vi "AutoBurn - BCU.vi"() -> ()   [LabVIEW 2018]
uses:
  <vilib>/Utility/config.llb/Read Key (String).vi
  <vilib>/Utility/config.llb/Write Key (String).vi
  <vilib>/Utility/file.llb/Read From Spreadsheet File (string).vi
  Settings/ControlCAN.dll
  <vilib>/Utility/config.llb/NI_LVConfig.lvlib
panel:
  out "?":bool
  in  "波特率 2":T1(ring)=enum."500Kbps"
  in  "错误输入（无错误）":errorcluster
  out "开始下载数据":u32
  out "开始下载数据":bool=TRUE
  out "耗时：":u32
  out "start":u32
  out "update flag":bool=TRUE
  in  "目标板类型":enum16{"BCU/主板", "BMU/从板"}(ring)
  out "Random":u32
  out "CRC16":u16 format="%x"
  out "进入烧录":bool
  out "boot模式应答计数":i32
  out "boot模式应答...成功":bool=TRUE
  out "总行数":i32
  in  "错误输入（无错误） 7":errorcluster caption="错误输入（无错误）"
  out "错误输出 18":errorcluster caption="错误输出"
  out "当前发送行":i32
  in  "错误输入（无错误） 6":errorcluster caption="错误输入（无错误）"
  out "错误输出 17":errorcluster caption="错误输出"
  in  "错误输入（无错误） 5":errorcluster caption="错误输入（无错误）"
  out "错误输出 16":errorcluster caption="错误输出"
  in  "错误输入（无错误） 4":errorcluster caption="错误输入（无错误）"
  out "错误输出 15":errorcluster caption="错误输出"
  in  "错误输入（无错误） 3":errorcluster caption="错误输入（无错误）"
  out "错误输出 14":errorcluster caption="错误输出"
  out "错误输出 13":errorcluster caption="错误输出"
  out "错误输出 12":errorcluster caption="错误输出"
  out "总电压":dbl
  out "Life":dbl
  out "返回类型":u32 format="%x"
  out "Info：":string
  in  "手动进入编程模式 2":bool
  out "T9":bool=TRUE
  out "T8":u8
  out "T7":bool=TRUE
  out "T6":bool=TRUE
  out "T5":bool=TRUE
  out "T4":bool=TRUE
  out "T3":bool=TRUE
  out "T2":bool=TRUE
  out "T1":bool=TRUE
  out "ID":u32 format="%x"
  out "错误输出 3":errorcluster caption="错误输出"
  in  "Monitor":bool
  out "校验":bool
  in  "请选择板号":u16(ring)=1 items=["BMU1"=1, "BMU2"=2, "BMU3"=3, "BMU4"=4, "BMU5"=5, "BMU6"=6, "BMU7"=7, "BMU8"=8, "BMU9"=9, "BMU10"=10, "BMU11"=11, "BMU12"=12, "BMU13"=13, "BMU14"=14, "BMU15"=15, "BMU16"=16, "BMU17"=17, "BMU18"=18, "BMU19"=19, "BMU20"=20]
  in  "手动进入编程模式":bool
  in  "板类型":enum16{"请选择板类型", "主板", "从板", "高压板"}(ring)=enum."主板"
  out "烧录结果":bool=TRUE
  out "擦除完成":bool
  out "进入烧录模式":bool
  out "MD5校验":bool
  out "进度":u8(slide) scale=0.0..100.0
  out "校验码实际值":string
  in  "校验码期望值":string
  in  "应用程序路径":path
  out "连接状态":bool=TRUE
  in  "类型":u32(ring)=4 items=["PCI5121"=1, "PCI9810"=2, "USBCAN1"=3, "USBCAN2"=4, "PCI9820"=5, "CAN232"=6, "PCI5110"=7, "CANLite(mini)"=8, "ISA9620"=9, "ISA5420"=10, "PC104CAN"=11, "CANET"=17, "DNP9810"=13, "USBCAN-E-U"=20, "USBCAN-2E-U"=21]
  in  "CAN路数":u32(ring) items=["0", "1"]
  in  "滤波方式":u8(ring) items=["Dual Filter", "Single Filter"]
  in  "工作方式":u8(ring) items=["Normal", "Listen Only"]
  in  "波特率":T1(ring)=enum."500Kbps"
  in  "设备索引":u32(ring) items=["0", "1", "2", "3", "4", "5", "6", "7", "8", "9", "10", "11", "12", "13", "14", "15", ""]
  in  "开始监控":bool
  out "CAN数据":bool
  out "Monitor_flag":bool
  out "PC端-协议类型 2":enum16{"TCP服务器Server", "TCP客户端Client"}(ring)
  out "通信端口:":u32
  out "CANET地址格式如：192.168.0.178":string
  out "发送数据长度":dbl
  out "发送的数据":i32[](array[numeric])
  in  "设备索引 4":u16(ring) items=["0", "1", "2", "3", "4", "5", "6", "7", "8", "9", "10", "11", "12", "13", "14", "15", ""]
  in  "CAN路数 4":u16(ring) items=["0", "1"]
  in  "设备类型 4":u16(ring)=4 items=["PCI5121"=1, "PCI9810"=2, "USBCAN1"=3, "USBCAN2"=4, "PCI9820"=5, "CAN232"=6, "PCI5110"=7, "CANLite(mini)"=8, "ISA9620"=9, "ISA5420"=10, "PC104CAN"=11, "CANETE"=12, "DNP9810"=13]
  out "Mode":bool
  in  "开始监控 2":bool
  out "大小":i32=426
  out "地址长度 2":u32=4
  out "数据长度 2":u32=64
  out "子字符串 2":string="9B2F9B349B399B3E9B439B499B4F9B559B5B9B619B679B6D9B739B799B7F7C7B"
  out "数据长度":u32=64
  out "地址长度":u32=4
  in  "设定":bool
  out "VCI_CAN_OBJ_T":T2 {"ID" format="%x"}
  out "子数组":string[](array[string])
  in  "从板号":dbl
  out "从板号2":dbl
  in  "读取":bool
  in  "停止 3":bool
  out "TEMP":bool
  out "CAN状态 2":bool
  out "VCI_CAN_OBJ_R":T2={"ID"=0, "TimeStamp"=0, "TimeFlag"=0, "SendType"=1, "RemoteFlag"=0, "ExternFlag"=0, "DataLen"=8, 0, 0, 0, 0, 0, 0, 0, 0, 0, 0, 0}
  in  "停止 2":bool
  out "接收":T2={"ID"=0, "TimeStamp"=61537964, "TimeFlag"=1, "SendType"=250, "RemoteFlag"=0, "ExternFlag"=0, "DataLen"=1, 255, 0, 0, 0, 0, 0, 0, 0, 0, 0, 124} {"ID" min=2 max=104373490 step=1 format="%x"; "TimeStamp" min=1962977793 max=3175728; "TimeFlag" min=1 max=0; "SendType" max=131 step=11; "RemoteFlag" min=52 max=6 step=1; "ExternFlag" max=0; "DataLen" min=1 max=170; "?" min=117 max=48 step=117; "?" min=48 max=0; "?" max=0; "?" min=2 max=0; "?" max=150 step=11; "?" min=52 max=6 step=1; "?" max=0; "?" min=1 max=170; "?" min=120 max=175; "?" max=12; "?" max=0}
  out "收到请求":bool=TRUE
  out "分配":bool
  out "设置中？ 2":bool
  in  "Boar_Type":bool
  out "temp1":bool
  out "设置中？":bool
  in  "总步骤":dbl=21.0
  in  "失败重测次数":dbl=3.0
  out "一键测试":bool
  out "测试结果":bool
  in  "行号":dbl=21.0
  in  "工作方式 2":u8(ring) items=["Normal", "Listen Only"]
  in  "设备类型 2":u16(ring)=4 items=["PCI5121"=1, "PCI9810"=2, "USBCAN1"=3, "USBCAN2"=4, "PCI9820"=5, "CAN232"=6, "PCI5110"=7, "CANLite(mini)"=8, "ISA9620"=9, "ISA5420"=10, "PC104CAN"=11, "CANETE"=12, "DNP9810"=13]
  in  "停止":bool
  out "CAN状态":bool=TRUE
  in  "监控":bool
  # "当前BMU信息"
  # "BootLoader_V1.0.0"
  # "注意：升级完成后系统需要重新上电才能正常运行！"
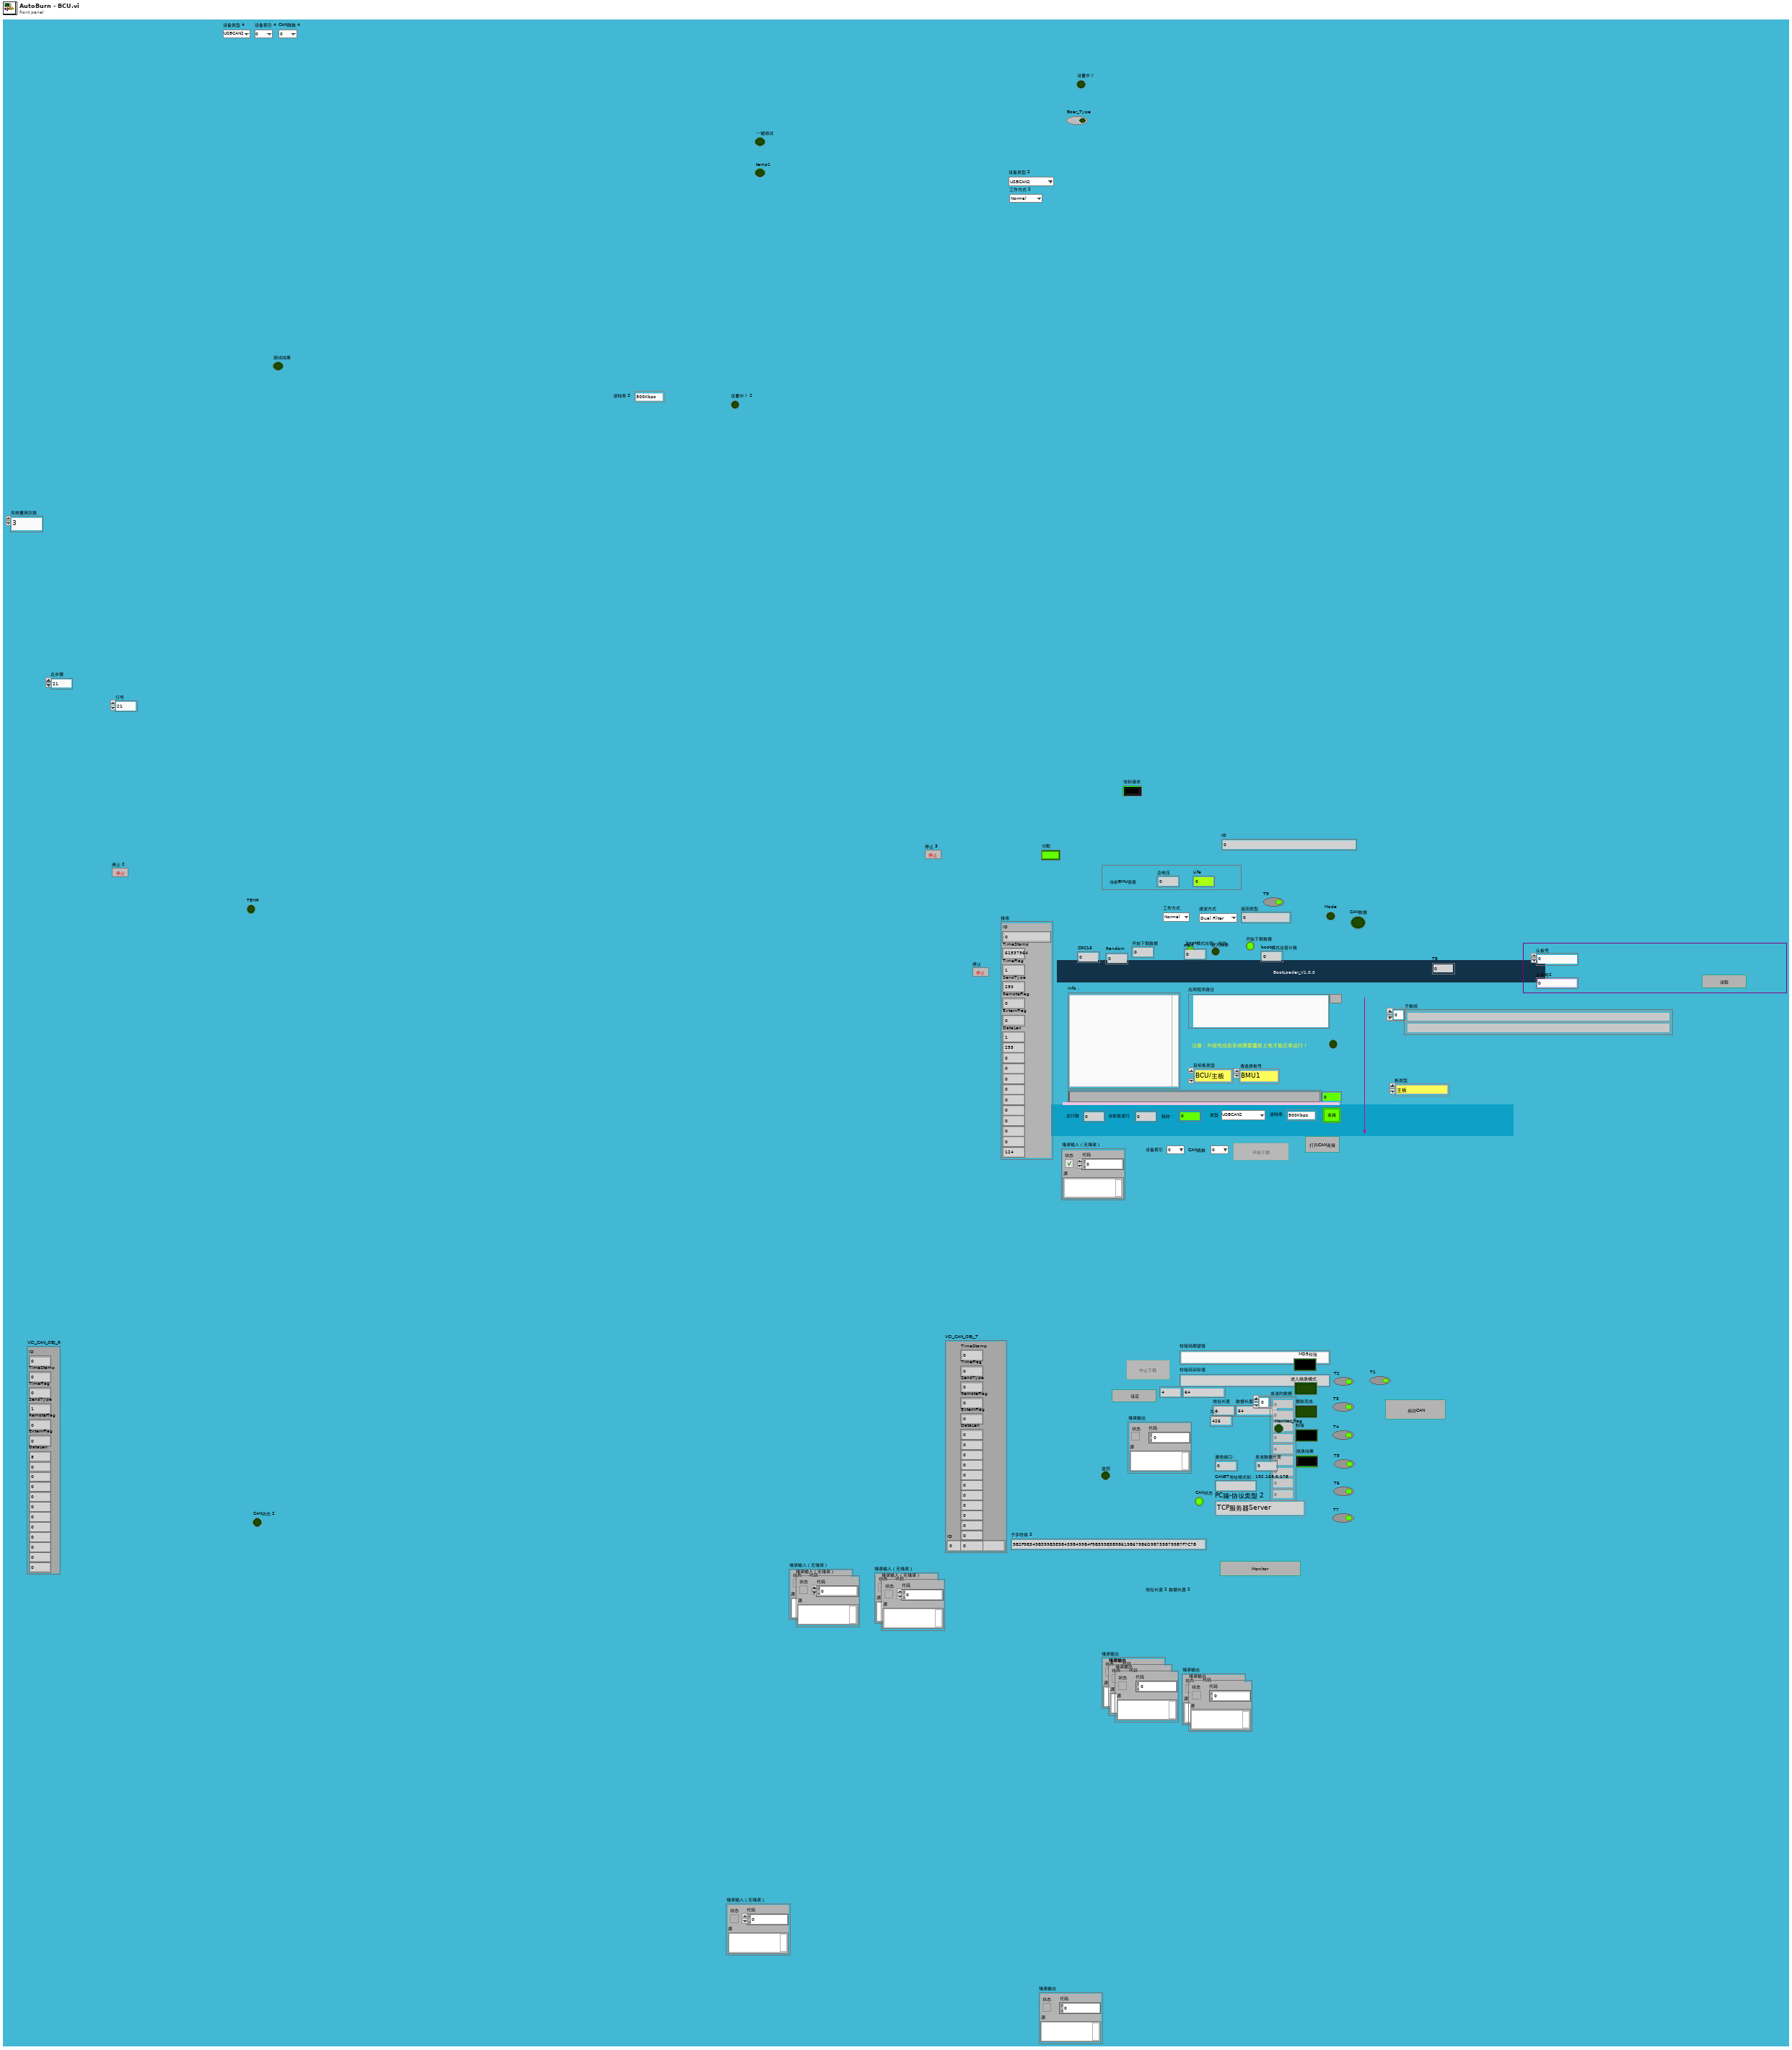
[diagram p1: front panel]
types:
  T1 = enum16{"5Kbps", "10Kbps", "20Kbps", "40Kbps", "50Kbps", "80Kbps", "100Kbps", "125Kbps", "200Kbps", "250Kbps", "400Kbps", "500Kbps", "666Kbps", "800Kbps", "1000Kbps"}
  T2 = cluster{"ID":u32, "TimeStamp":u32, "TimeFlag":u8, "SendType":u8, "RemoteFlag":u8, "ExternFlag":u8, "DataLen":u8, u8, u8, u8, u8, u8, u8, u8, u8, u8, u8, u8}
  T3 = enum8{"Enabled", "Disabled", "Disabled and Grayed Out"}
  T4 = typedef "NI_LVConfig.lvlib/Config Data RefNum.ctl" = refnum<k1>
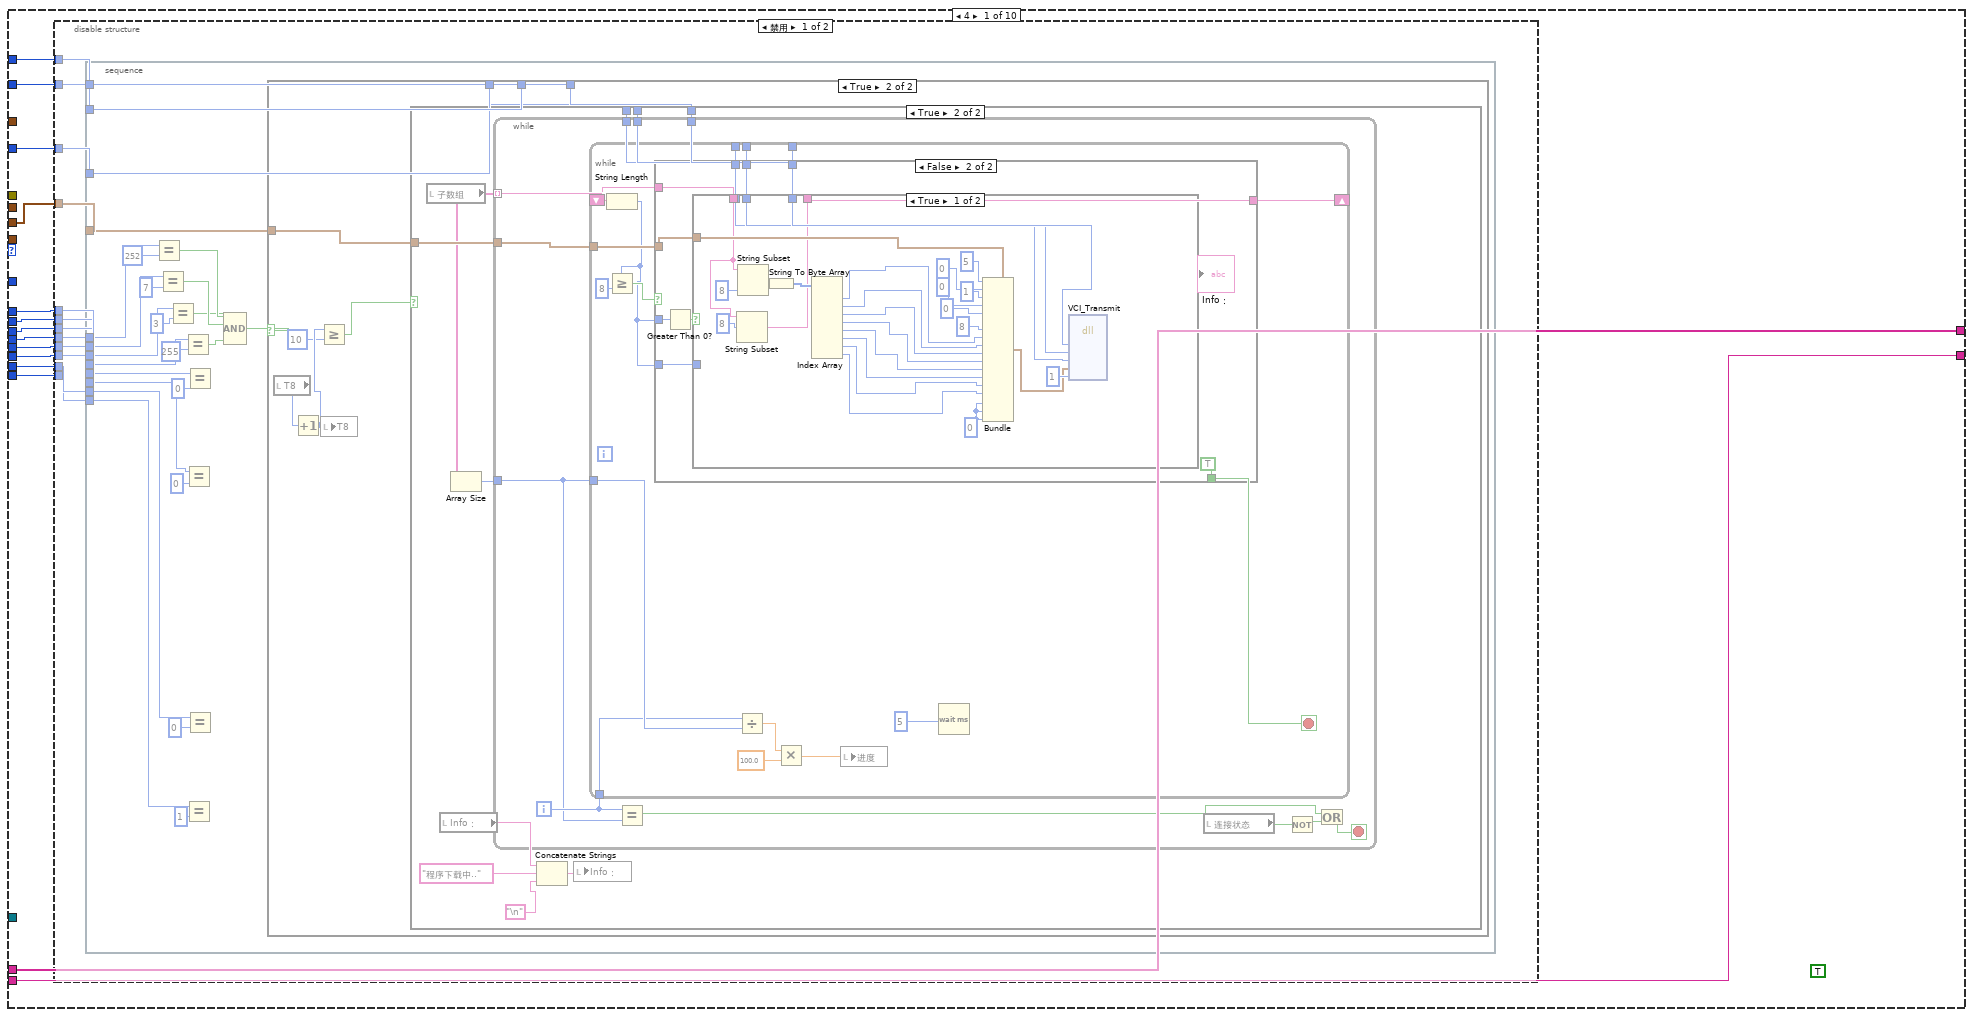
[diagram p3: hidden frame]
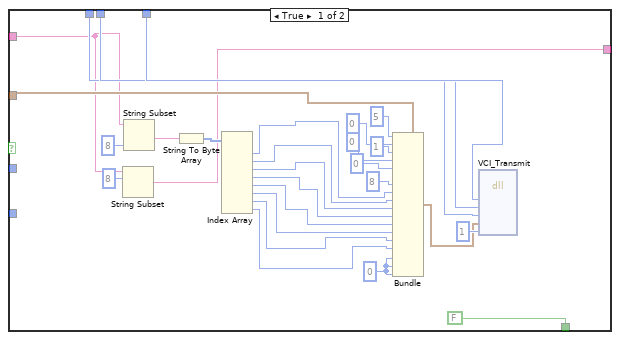
[diagram p6: hidden frame]
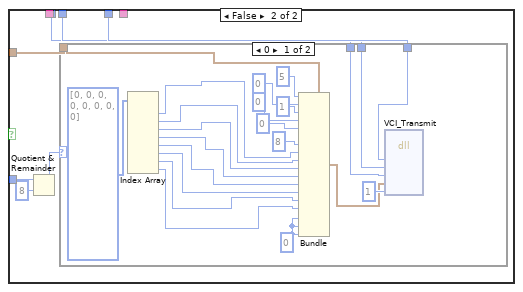
[diagram p7: hidden frame]
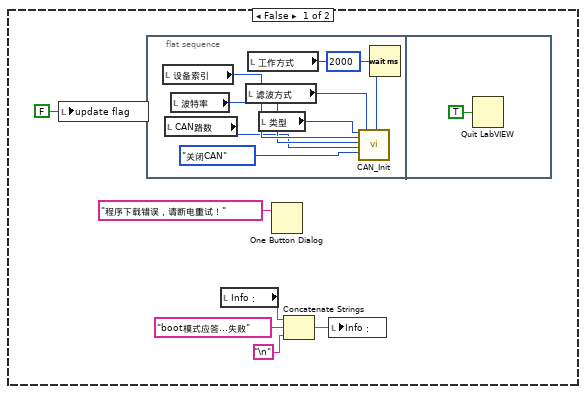
[diagram p10: hidden frame]
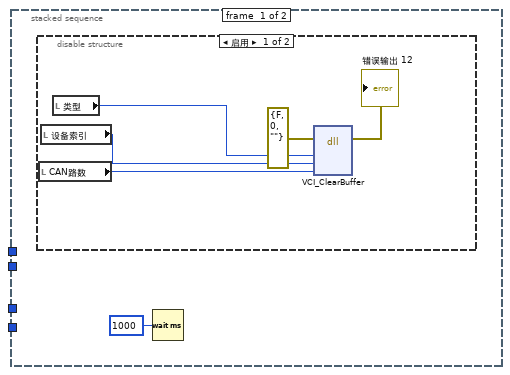
[diagram p11: hidden frame]
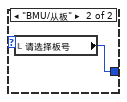
[diagram p13: hidden frame]
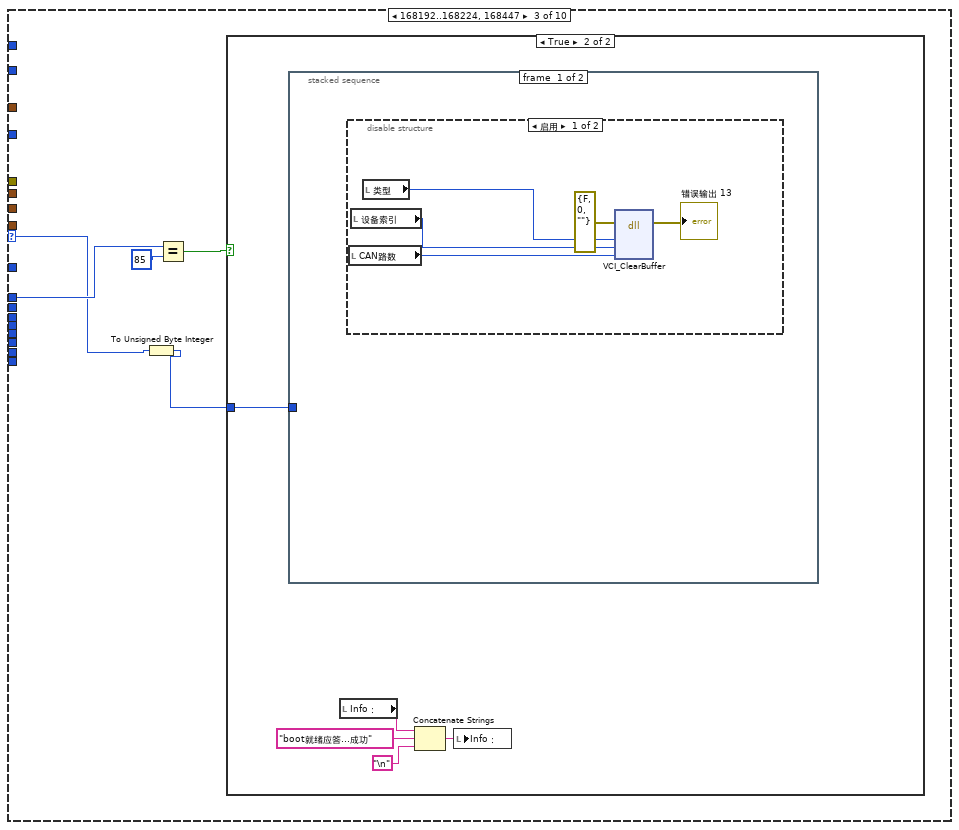
[diagram p14: hidden frame]
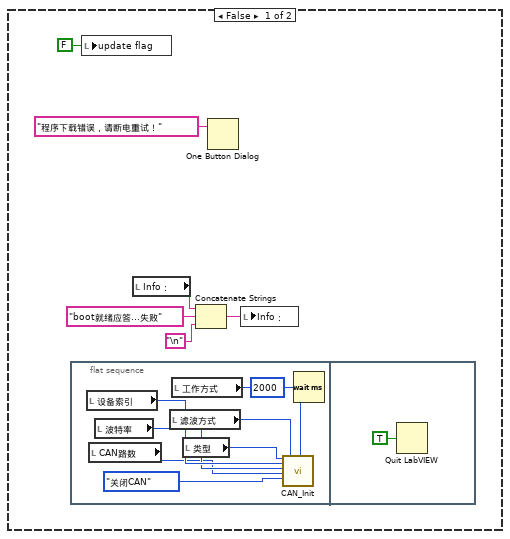
[diagram p15: hidden frame]
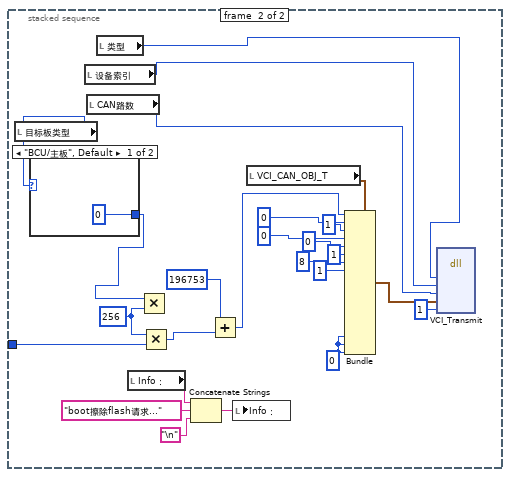
[diagram p17: hidden frame]
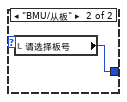
[diagram p18: hidden frame]
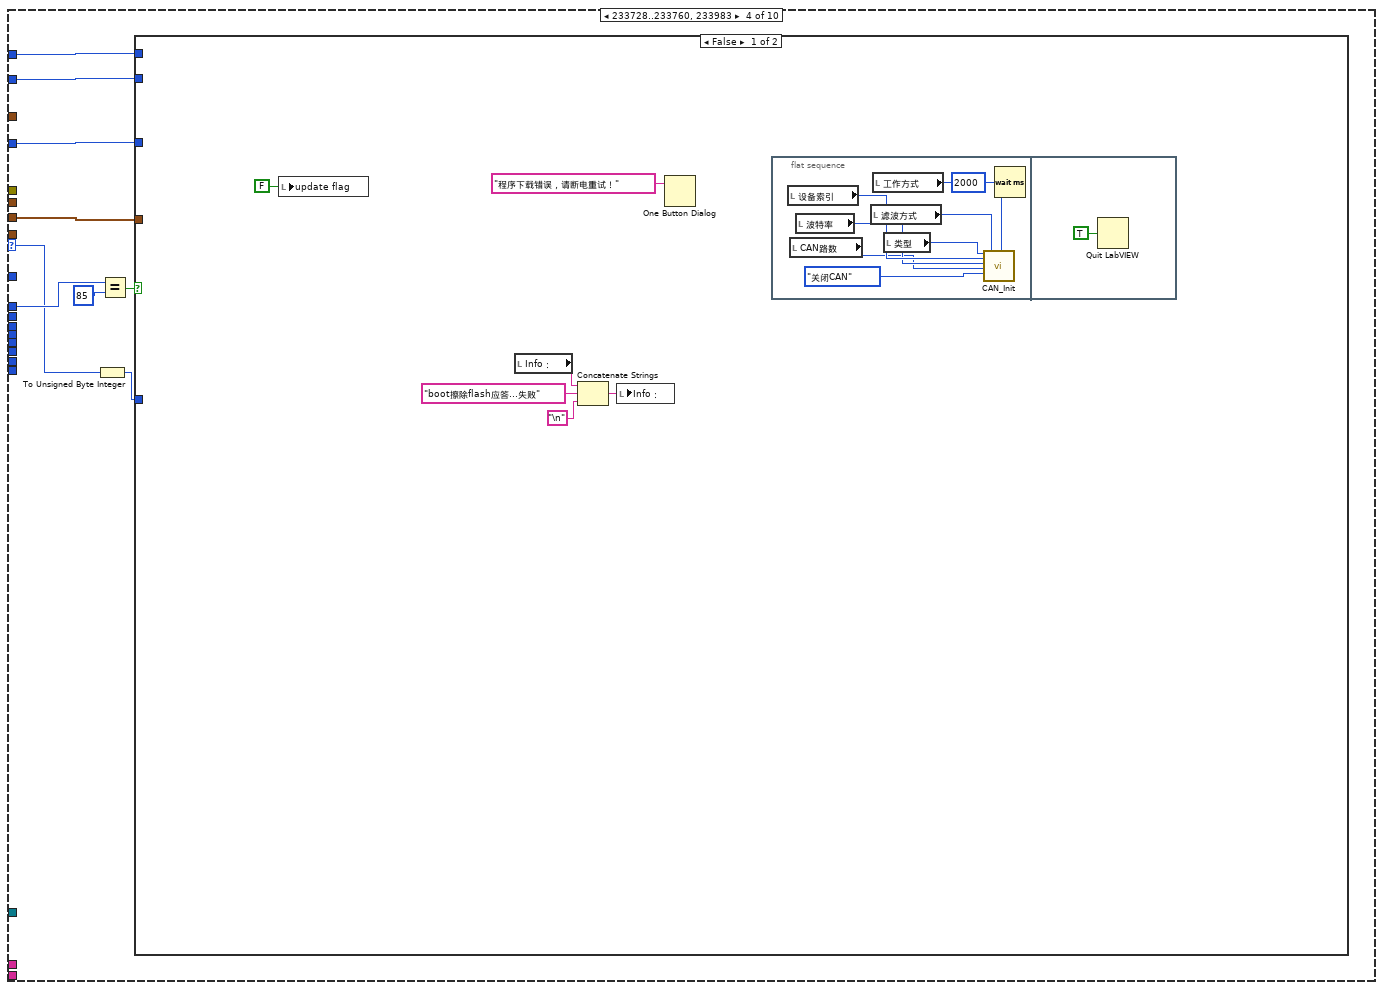
[diagram p19: hidden frame]
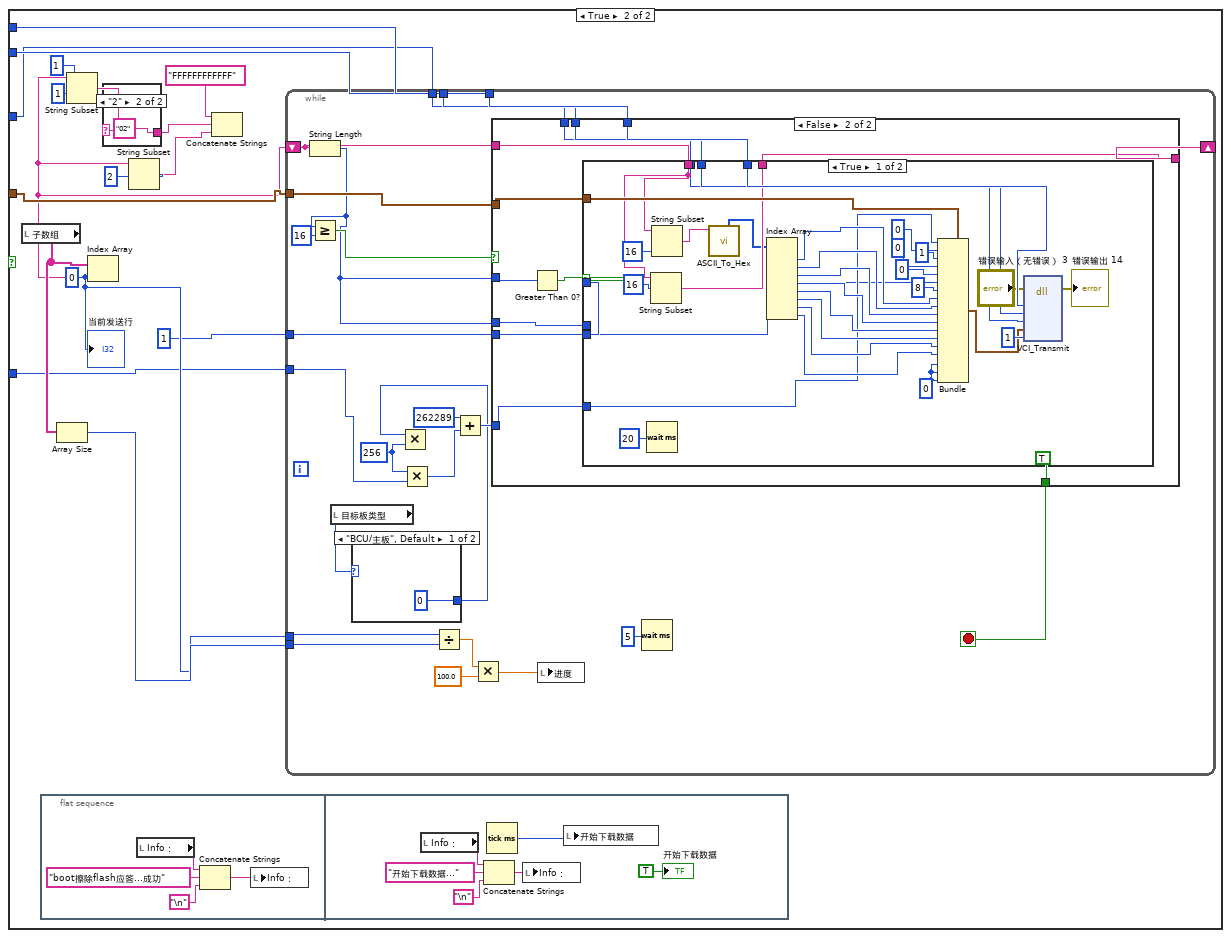
[diagram p20: hidden frame]
diagram:
  (unwired) u32 0
  (unwired) u32 255
  w21 = "" ("布尔文本.文本")
  w22 = cluster{u32, u32}[] [{0, 0}] ("颜色[4]")
  w29 = "" ("校验码期望值")
  w37 = FALSE ("进入烧录模式")
  n1 = local write "TEMP"(FALSE ("TEMP")) -> ()
  n2 = local read "VCI_CAN_OBJ_R"() -> (w19:T2)
  n3 = local write "校验码期望值"(w29) -> ()
  n4 = local write "校验码实际值"(w29) -> ()
  n5 = property on="校验" class="Bool (strict)"("Colors [4]"=w22, "BoolText.Text"=w21) -> ()  [unwired: 2 in, 2 out]
  n6 = Obtain Queue(name (unnamed)="CAN1" ("名称（未命名）"), element data type=w19, error in (no error)="错误输入（无错误）") -> (queue out=w20:refnum<queue>, error out=w7:errorcluster)  [unwired: 2 in, 1 out]
  n7 = property on="烧录结果" class="Bool (strict)"("Colors [4]"=w22, "BoolText.Text"=w21) -> ()  [unwired: 2 in, 2 out]
  n8 = Initialize Array("", 1 ("维数大小")) -> (w33:string[])
  n9 = local write "连接状态"(FALSE ("连接状态")) -> ()
  n10 = local write "boot模式应答...成功"(FALSE ("boot模式应答...成功")) -> ()
  n11 = local write "开始下载数据"(u32 0 ("开始下载数据")) -> ()
  n12 = local write "耗时："(u32 0 ("耗时：")) -> ()
  n13 = property on="请选择板号" class="Ring (strict)"("Visible"=TRUE ("可见")) -> ()  [unwired: 2 in, 2 out]
  n14 = local write "耗时："(u32 0 ("耗时：")) -> ()
  n15 = while {
    tunnel: w20 -> [w44]
    shift-right: [w47] -> _
    shift-left: w33 -> [w48]
    shift-right: [w45] -> _
    shift-left: "" -> [w46]
    tunnel: w7 -> [w43]
    stop <- "停止 3" stop-if-true
    n16 = local read "update flag"() -> (w40:bool)
    n17 = Dequeue Element(queue=w44, error in (no error)=w43) -> (element=w41:T2, error out=w42:errorcluster)  [unwired: 1 in, 2 out]
    n18 = case shown="True" w40 {
      tunnel: w48 -> [_ w67]
      tunnel: [_ w66] -> w47
      tunnel: w46 -> [_ w65]
      tunnel: [_ w64] -> w45
      tunnel: w44 -> [_ w62]
      tunnel: w42 -> [_ w61]
      tunnel: w41 -> [_ w60]
      frame False {
      }
      frame True {
        n19 = local read "VCI_CAN_OBJ_T"() -> (w70:T2)
        n20 = local read "CAN路数"() -> (w68:u32)
        n21 = Unbundle(w60) -> ("ID"=w59:u32, w58:u8, w57:u8, w56:u8, w55:u8, w54:u8, w53:u8, w52:u8, w51:u8)  [unwired: 9 out]
        n22 = local read "类型"() -> (w69:u32)
        n23 = local read "设备索引"() -> (w50:u32)
        n24 = case shown="19100..19120, 191FF" w59 {
          selector: w59 -> [_ w266 w348 w404 w592 _ _ _ _ w1335]
          tunnel: w60 -> [_ _ _ _ _ _ _ _ _ _]
          tunnel: w70 -> [w84 _ _ w408 w596 w814 w879 _ w1115 _]
          tunnel: w69 -> [w83 _ _ w407 w595 w813 w881 w1009 w1123 _]
          tunnel: w50 -> [w82 _ _ w406 w594 w812 w880 w1008 w1122 _]
          tunnel: w68 -> [w81 _ _ w405 w593 w811 w878 w1007 w1121 _]
          tunnel: w67 -> [w80 _ _ _ _ w810 w883 w1006 w1117 w1337]
          tunnel: [w80 _ _ _ _ w810 w882 w1006 w1118 w1337] -> w66
          tunnel: w65 -> [w79 _ _ _ _ w809 w877 w1011 w1119 w1336]
          tunnel: [w79 _ _ _ _ w809 w876 w1010 w1120 w1336] -> w64
          tunnel: "板类型" -> [_ _ _ _ _ _ w875 w1005 w1116 _]
          tunnel: w62 -> [_ _ _ _ _ w808 w874 w1004 w1114 _]
          tunnel: w61 -> [_ _ _ _ _ _ _ _ _ _]
          tunnel: w60 -> [_ _ _ _ _ _ _ w995 _ _]
          tunnel: w60 -> [_ _ _ _ _ _ _ _ w1113 _]
          tunnel: w58 -> [w78 w269 w350 w411 _ _ _ _ _ _]
          tunnel: w57 -> [w77 w264 _ _ _ _ _ _ _ _]
          tunnel: w56 -> [w76 w263 _ _ w590 _ _ _ _ _]
          tunnel: w55 -> [w75 w262 _ _ _ _ _ _ _ _]
          tunnel: w54 -> [w74 w261 _ _ _ _ _ _ _ _]
          tunnel: w53 -> [w73 _ _ _ _ _ _ _ _ _]
          tunnel: w52 -> [w72 _ _ _ _ _ _ _ _ w1331]
          tunnel: w51 -> [w71 _ _ _ _ _ _ _ _ w1330]
          frame 4 {
            (unwired) TRUE
            n25 = disable-structure shown="禁用" {
              disable-tunnel: w84 -> [w96 _]
              disable-tunnel: w83 -> [w95 _]
              disable-tunnel: w82 -> [w94 _]
              disable-tunnel: w81 -> [w93 _]
              disable-tunnel: w78 -> [w92 _]
              disable-tunnel: w77 -> [w91 _]
              disable-tunnel: w76 -> [w90 _]
              disable-tunnel: w75 -> [w89 _]
              disable-tunnel: w74 -> [w88 _]
              disable-tunnel: w73 -> [w87 _]
              disable-tunnel: w72 -> [w86 _]
              disable-tunnel: w71 -> [w85 _]
              frame Disabled {
                n26 = stacked-sequence {
                  tunnel: w96 -> [w121]
                  tunnel: w95 -> [w120]
                  tunnel: w94 -> [w119]
                  tunnel: w93 -> [w118]
                  tunnel: w92 -> [w117]
                  tunnel: w91 -> [w116]
                  tunnel: w90 -> [w115]
                  tunnel: w89 -> [w114]
                  tunnel: w88 -> [w113]
                  tunnel: w87 -> [w112]
                  tunnel: w86 -> [w111]
                  tunnel: w85 -> [w110]
                  frame #0 {
                    n27 = Equal?(x=w117, y=u8 252) -> (x = y?=w101:bool)
                    n28 = Equal?(x=w116, y=u8 7) -> (x = y?=w100:bool)
                    n29 = Equal?(x=w115, y=u8 3) -> (x = y?=w99:bool)
                    n30 = Equal?(x=w114, y=u8 255) -> (x = y?=w98:bool)
                    n31 = Equal?(x=w112, y=u8 0) -> ()  [unwired: 1 out]
                    n32 = Equal?(x=w110, y=u8 1) -> ()  [unwired: 1 out]
                    n33 = Equal?(x=w113, y=u8 0) -> ()  [unwired: 1 out]
                    n34 = Equal?(x=w111, y=u8 0) -> ()  [unwired: 1 out]
                    n35 = Compound Arithmetic op=AND(w101, w100, w99, w98) -> (w97:bool)
                    n36 = case shown="True" w97 {
                      tunnel: w121 -> [_ w129]
                      tunnel: w120 -> [_ w128]
                      tunnel: w119 -> [_ w127]
                      tunnel: w118 -> [_ w126]
                      frame False {
                      }
                      frame True {
                        n37 = local read "T8"() -> (w125:u8)
                        n38 = Increment(x=w125) -> (x+1=w124:u8)
                        n39 = Greater Or Equal?(x=w124, y=u8 10) -> (x >= y?=w122:bool)
                        n40 = local write "T8"(w124) -> ()
                        n41 = case shown="True" w122 {
                          tunnel: w129 -> [_ w139]
                          tunnel: w128 -> [_ w138]
                          tunnel: w127 -> [_ w137]
                          tunnel: w126 -> [_ w136]
                          frame False {
                          }
                          frame True {
                            n42 = local read "子数组"() -> (w135:string[])
                            n43 = local read "Info："() -> (w131:string)
                            n44 = Array Size(array=w135) -> (size(s)=w134:i32)
                            n45 = while {
                              tunnel: w139 -> [w150]
                              tunnel: w138 -> [w149]
                              tunnel: w137 -> [w148]
                              tunnel: w136 -> [w147]
                              tunnel: w135 -> [w146] mode=indexing
                              tunnel: w134 -> [w143]
                              i -> [w144]
                              stop <- w142 stop-if-true
                              n46 = while {
                                tunnel: w150 -> [w166]
                                tunnel: w149 -> [w165]
                                tunnel: w148 -> [w164]
                                tunnel: w147 -> [w163]
                                shift-right: [w158] -> _
                                shift-left: w146 -> [w159]
                                tunnel: w143 -> [w156]
                                tunnel: w144 -> [w152]
                                stop <- w151 stop-if-true
                                n47 = String Length(string=w159) -> (length=w157:i32)
                                n48 = Greater Or Equal?(x=w157, y=8) -> (x >= y?=w160:bool)
                                n49 = case shown="False" w160 {
                                tunnel: w166 -> [w194 w204]
                                tunnel: w165 -> [w193 w203]
                                tunnel: w164 -> [w192 w202]
                                tunnel: w163 -> [w191 w201]
                                tunnel: w159 -> [w180 w200]
                                tunnel: [w168 w199] -> w158
                                tunnel: [FALSE TRUE] -> w151
                                tunnel: w157 -> [_ w197]
                                tunnel: w157 -> [_ w195]
                                frame True {
                                w187 = u8 0 ("元素")
                                n50 = String Subset(string=w180, offset (0)=8 ("偏移量(0)")) -> (substring=w168:string)  [unwired: 1 in]
                                n51 = String Subset(string=w180, length (rest)=8 ("长度（剩余）")) -> (substring=w178:string)  [unwired: 1 in]
                                n52 = String To Byte Array(string=w178) -> (unsigned byte array=w177:u8[])
                                n53 = Index Array(array=w177) -> (element #1=w176:u8, element #2=w175:u8, element #3=w174:u8, element #4=w173:u8, element #5=w172:u8, element #6=w171:u8, element #7=w170:u8, element #8=w169:u8)  [unwired: 8 in]
                                n54 = Bundle(cluster=w194, "ID"=u32 5, "TimeStamp"=u8 0 ("RemoteFlag"), "TimeFlag"=u8 1, "SendType"=u8 0 ("DataLen"), "RemoteFlag"=u8 0, "DataLen"=u8 8, w176, w175, w174, w173, w172, w171, w170, w169, w187, w187, w187) -> (w182:T2)  [unwired: 1 in]
                                n55 = dll-call lib="PTH2{abs DPCTools2.sourceSNV-AutoTestV1.0.0ASettingsSEQEditDriver平台BCUAutoBurnSettingsControlCAN.dll" fn="VCI_Transmit"("DeviceType"=w193, "DeviceInd"=w192, "CANInd"=w191, "pSend"=w182, "Len"=u32 1) -> ()  [unwired: 5 in, 6 out]
                                }
                                frame False {
                                n56 = Greater Than 0?(x=w197) -> (x > 0?=w196:bool)
                                n57 = case shown="True" w196 {
                                tunnel: w204 -> [w231 w238]
                                tunnel: w203 -> [w230 w237]
                                tunnel: w202 -> [w229 w236]
                                tunnel: w201 -> [w228 w235]
                                tunnel: w200 -> [w217 _]
                                tunnel: [w206 _] -> w199
                                tunnel: w195 -> [_ w233]
                                frame True {
                                w224 = u8 0 ("元素")
                                n58 = String Subset(string=w217, offset (0)=8 ("偏移量(0)")) -> (substring=w206:string)  [unwired: 1 in]
                                n59 = String Subset(string=w217, length (rest)=8 ("长度（剩余）")) -> (substring=w216:string)  [unwired: 1 in]
                                n60 = String To Byte Array(string=w216) -> (unsigned byte array=w215:u8[])
                                n61 = Index Array(array=w215) -> (element #1=w214:u8, element #2=w213:u8, element #3=w212:u8, element #4=w211:u8, element #5=w210:u8, element #6=w209:u8, element #7=w208:u8, element #8=w207:u8)  [unwired: 8 in]
                                n62 = Bundle(cluster=w231, "ID"=u32 5, "TimeStamp"=u8 0 ("RemoteFlag"), "TimeFlag"=u8 1, "SendType"=u8 0 ("DataLen"), "RemoteFlag"=u8 0, "DataLen"=u8 8, w214, w213, w212, w211, w210, w209, w208, w207, w224, w224, w224) -> (w219:T2)  [unwired: 1 in]
                                n63 = dll-call lib="PTH2{abs DPCTools2.sourceSNV-AutoTestV1.0.0ASettingsSEQEditDriver平台BCUAutoBurnSettingsControlCAN.dll" fn="VCI_Transmit"("DeviceType"=w230, "DeviceInd"=w229, "CANInd"=w228, "pSend"=w219, "Len"=u32 1) -> ()  [unwired: 5 in, 6 out]
                                }
                                frame False {
                                n64 = Quotient & Remainder(x=w233, y=8) -> (x-y*floor(x/y)=w232:i32)  [unwired: 1 out]
                                n65 = case shown="0" w232 {
                                tunnel: w238 -> [w260 _]
                                tunnel: w237 -> [w259 _]
                                tunnel: w236 -> [w258 _]
                                tunnel: w235 -> [w257 _]
                                frame 0 {
                                w253 = u8 0 ("元素")
                                n66 = Index Array(array=u8[] [0, 0, 0, 0, 0, 0, 0, 0] ("数组")) -> (element #1=w247:u8, element #2=w246:u8, element #3=w245:u8, element #4=w244:u8, element #5=w243:u8, element #6=w242:u8, element #7=w241:u8, element #8=w240:u8)  [unwired: 8 in]
                                n67 = Bundle(cluster=w260, "ID"=u32 5, "TimeStamp"=u8 0 ("RemoteFlag"), "TimeFlag"=u8 1, "SendType"=u8 0 ("DataLen"), "RemoteFlag"=u8 0, "DataLen"=u8 8, w247, w246, w245, w244, w243, w242, w241, w240, w253, w253, w253) -> (w248:T2)  [unwired: 1 in]
                                n68 = dll-call lib="PTH2{abs DPCTools2.sourceSNV-AutoTestV1.0.0ASettingsSEQEditDriver平台BCUAutoBurnSettingsControlCAN.dll" fn="VCI_Transmit"("DeviceType"=w259, "DeviceInd"=w258, "CANInd"=w257, "pSend"=w248, "Len"=u32 1) -> ()  [unwired: 5 in, 6 out]
                                }
                                frame 1, Default {
                                }
                                }
                                }
                                }
                                }
                                }
                                n69 = Divide(x=w152, y=w156) -> (x/y=w155:dbl)
                                n70 = Multiply(x=w155, y=100.0) -> (x*y=w153:dbl)
                                n71 = local write "进度"(w153) -> ()
                                n72 = Wait (ms)(milliseconds to wait=u32 5 ("等待时间（毫秒）")) -> ()  [unwired: 1 out]
                              }
                              n73 = Equal?(x=w144, y=w143) -> (x = y?=w140:bool)
                              n74 = local read "连接状态"() -> (w145:bool)
                              n75 = Not(x=w145) -> (.not. x?=w141:bool)
                              n76 = Or(x=w140, y=w141) -> (x .or. y?=w142:bool)
                            }
                            n77 = Concatenate Strings(w131, "程序下载中.." ("字符串"), "\n") -> (w130:string)
                            n78 = local write "Info："(w130) -> ()
                          }
                        }
                      }
                    }
                  }
                }
              }
              frame Enabled {
              }
            }
          }
          frame 102656..102688, 102911 {
            n79 = To Unsigned Byte Integer(number=w266) -> (unsigned 8bit integer=w265:u8)
            n80 = Equal?(x=w269, y=u8 85) -> (x = y?=w268:bool)
            n81 = case shown="True" w268 {
              tunnel: w265 -> [_ w301]
              tunnel: w264 -> [_ w298]
              tunnel: w263 -> [_ w296]
              tunnel: w262 -> [_ w297]
              tunnel: w261 -> [_ w295]
              frame False {
                n82 = local write "update flag"(FALSE ("update flag")) -> ()
                n83 = flat-sequence {
                  frame #0 {
                    n84 = local read "设备索引"() -> (w282:u32)
                    n85 = local read "CAN路数"() -> (w280:u32)
                    n86 = local read "波特率"() -> (w281:T1)
                    n87 = local read "滤波方式"() -> (w279:u8)
                    n88 = local read "工作方式"() -> (w278:u8)
                    n89 = local read "类型"() -> (w283:u32)
                    n90 = call "CAN_Init.vi"("设备类型"=w283, "设备索引"=w282, "波特率"=w281, "CAN路数"=w280, "操作类型"=enum16{"初始化CAN", "关闭CAN"}."关闭CAN", "滤波方式"=w279, "工作方式"=w278) -> ()  [unwired: 11 in, 2 out]
                    n91 = Wait (ms)(milliseconds to wait=u32 2000 ("等待时间（毫秒）")) -> ()  [unwired: 1 out]
                  }
                  frame #1 {
                    n92 = Quit LabVIEW(quit? (T)=TRUE ("退出？(T)")) -> ()
                  }
                }
                n93 = local read "Info："() -> (w272:string)
                n94 = One Button Dialog(message="程序下载错误，请断电重试！" ("消息")) -> ()  [unwired: 1 in, 1 out]
                n95 = Concatenate Strings(w272, "boot模式应答...失败" ("字符串"), "\n") -> (w275:string)
                n96 = local write "Info："(w275) -> ()
              }
              frame True {
                n97 = Join Numbers(hi=w298, lo=w297) -> ((hi.lo)=w294:u16)
                n98 = Join Numbers(hi=w295, lo=w296) -> ((hi.lo)=w293:u16)
                n99 = Join Numbers(hi=w294, lo=w293) -> ((hi.lo)=w292:u32)
                n100 = Not(x=w292) -> (.not. x?=w291:u32)
                "Random" <- w291
                n101 = Split Number(x=w291) -> (hi(x)=w290:u16, lo(x)=w289:u16)
                n102 = Split Number(x=w290) -> (hi(x)=w288:u8, lo(x)=w287:u8)
                n103 = Split Number(x=w289) -> (hi(x)=w286:u8, lo(x)=w285:u8)
                n104 = stacked-sequence {
                  tunnel: w301 -> [_ w322]
                  tunnel: w288 -> [_ w317]
                  tunnel: w287 -> [_ w316]
                  tunnel: w286 -> [_ w315]
                  tunnel: w285 -> [_ w314]
                  frame #0 {
                    n105 = disable-structure shown="启用" {
                      frame Enabled {
                        n106 = local read "CAN路数"() -> (w309:u32)
                        n107 = local read "设备索引"() -> (w310:u32)
                        n108 = local read "类型"() -> (w311:u32)
                        n109 = dll-call lib="PTH2{abs DPCTools2.sourceSNV-AutoTestV1.0.0ASettingsSEQEditDriver平台BCUAutoBurnSettingsControlCAN.dll" fn="VCI_ClearBuffer" label="VCI_Clearbuffer"(error in=errorcluster {"status"=FALSE, "code"=0, "source"=""} ("错误输入（无错误）"), "DeviceType"=w311, "DeviceInd"=w310, "CANInd"=w309) -> (error out=→"错误输出 12":errorcluster)  [unwired: 3 in, 4 out]
                      }
                      frame Disabled {
                      }
                    }
                    n110 = Wait (ms)(milliseconds to wait=u32 1000 ("等待时间（毫秒）")) -> ()  [unwired: 1 out]
                  }
                  frame #1 {
                    w323 = u16 256 ("y")
                    w338 = u8 0 ("元素")
                    n111 = local read "目标板类型"() -> (w313:enum16{"BCU/主板", "BMU/从板"})
                    n112 = case shown="\"BCU/主板\", Default" w313 {
                      tunnel: [u16 0 ("请选择板号") w345] -> w312
                      frame "BCU/主板", Default {
                      }
                      frame "BMU/从板" {
                        n113 = local read "请选择板号"() -> (w345:u16)
                      }
                    }
                    n114 = local read "设备索引"() -> (w333:u32)
                    n115 = local read "CAN路数"() -> (w332:u32)
                    n116 = local read "类型"() -> (w334:u32)
                    n117 = Multiply(x=w312, y=w323) -> ()  [unwired: 1 out]
                    n118 = Multiply(x=w323, y=w322) -> (x*y=w321:u16)
                    n119 = local read "Info："() -> (w327:string)
                    n120 = Add(x=u32 131217 ("ID"), y=w321) -> (x+y=w328:u32)
                    n121 = local read "VCI_CAN_OBJ_T"() -> (w331:T2)
                    n122 = local read "CRC16"() -> (w320:u16)
                    n123 = Concatenate Strings(w327, "boot就绪查询..." ("字符串"), "\n") -> (w324:string)
                    n124 = Split Number(x=w320) -> (hi(x)=w318:u8, lo(x)=w319:u8)
                    n125 = local write "Info："(w324) -> ()
                    n126 = Bundle(cluster=w331, "ID"=w328, "TimeStamp"=u8 0 ("RemoteFlag"), "TimeFlag"=u8 1, "SendType"=u8 0 ("DataLen"), "RemoteFlag"=u8 0, "ExternFlag"=u8 1, "DataLen"=u8 8, u8 1 ("元素"), w317, w316, w315, w314, w318, w319, w338, w338, w338) -> (w335:T2)  [unwired: 1 in]
                    n127 = dll-call lib="PTH2{abs DPCTools2.sourceSNV-AutoTestV1.0.0ASettingsSEQEditDriver平台BCUAutoBurnSettingsControlCAN.dll" fn="VCI_Transmit"("DeviceType"=w334, "DeviceInd"=w333, "CANInd"=w332, "pSend"=w335, "Len"=u32 1) -> ()  [unwired: 5 in, 6 out]
                  }
                }
                n128 = local read "Info："() -> (w302:string)
                n129 = local write "进入烧录"(FALSE ("进入烧录")) -> ()
                n130 = Concatenate Strings(w302, "boot模式应答...成功" ("字符串"), "\n") -> (w305:string)
                n131 = local write "Info："(w305) -> ()
                "boot模式应答...成功" <- TRUE
              }
            }
          }
          frame 168192..168224, 168447 {
            n132 = To Unsigned Byte Integer(number=w348) -> (unsigned 8bit integer=w347:u8)
            n133 = Equal?(x=w350, y=u8 85) -> (x = y?=w346:bool)
            n134 = case shown="True" w346 {
              tunnel: w347 -> [_ w370]
              frame False {
                n135 = flat-sequence {
                  frame #0 {
                    n136 = local read "设备索引"() -> (w363:u32)
                    n137 = local read "CAN路数"() -> (w361:u32)
                    n138 = local read "波特率"() -> (w362:T1)
                    n139 = local read "滤波方式"() -> (w360:u8)
                    n140 = local read "工作方式"() -> (w359:u8)
                    n141 = local read "类型"() -> (w364:u32)
                    n142 = call "CAN_Init.vi"("设备类型"=w364, "设备索引"=w363, "波特率"=w362, "CAN路数"=w361, "操作类型"=enum16{"初始化CAN", "关闭CAN"}."关闭CAN", "滤波方式"=w360, "工作方式"=w359) -> ()  [unwired: 11 in, 2 out]
                    n143 = Wait (ms)(milliseconds to wait=u32 2000 ("等待时间（毫秒）")) -> ()  [unwired: 1 out]
                  }
                  frame #1 {
                    n144 = Quit LabVIEW(quit? (T)=TRUE ("退出？(T)")) -> ()
                  }
                }
                n145 = local write "update flag"(FALSE ("update flag")) -> ()
                n146 = local read "Info："() -> (w353:string)
                n147 = Concatenate Strings(w353, "boot就绪应答...失败" ("字符串"), "\n") -> (w356:string)
                n148 = One Button Dialog(message="程序下载错误，请断电重试！" ("消息")) -> ()  [unwired: 1 in, 1 out]
                n149 = local write "Info："(w356) -> ()
              }
              frame True {
                n150 = stacked-sequence {
                  tunnel: w370 -> [_ w379]
                  frame #0 {
                    n151 = disable-structure shown="启用" {
                      frame Enabled {
                        n152 = local read "CAN路数"() -> (w373:u32)
                        n153 = local read "设备索引"() -> (w374:u32)
                        n154 = local read "类型"() -> (w375:u32)
                        n155 = dll-call lib="PTH2{abs DPCTools2.sourceSNV-AutoTestV1.0.0ASettingsSEQEditDriver平台BCUAutoBurnSettingsControlCAN.dll" fn="VCI_ClearBuffer" label="VCI_Clearbuffer"(error in=errorcluster {"status"=FALSE, "code"=0, "source"=""} ("错误输入（无错误）"), "DeviceType"=w375, "DeviceInd"=w374, "CANInd"=w373) -> (error out=→"错误输出 13":errorcluster)  [unwired: 3 in, 4 out]
                      }
                      frame Disabled {
                      }
                    }
                  }
                  frame #1 {
                    w380 = u16 256 ("y")
                    w395 = u8 0 ("元素")
                    n156 = local read "目标板类型"() -> (w377:enum16{"BCU/主板", "BMU/从板"})
                    n157 = case shown="\"BCU/主板\", Default" w377 {
                      tunnel: [u16 0 ("请选择板号") w402] -> w376
                      frame "BCU/主板", Default {
                      }
                      frame "BMU/从板" {
                        n158 = local read "请选择板号"() -> (w402:u16)
                      }
                    }
                    n159 = local read "设备索引"() -> (w390:u32)
                    n160 = local read "CAN路数"() -> (w389:u32)
                    n161 = local read "类型"() -> (w391:u32)
                    n162 = local read "Info："() -> (w381:string)
                    n163 = Multiply(x=w376, y=w380) -> ()  [unwired: 1 out]
                    n164 = Multiply(x=w380, y=w379) -> (x*y=w378:u16)
                    n165 = Concatenate Strings(w381, "boot擦除flash请求..." ("字符串"), "\n") -> (w384:string)
                    n166 = Add(x=u32 196753 ("ID"), y=w378) -> (x+y=w385:u32)
                    n167 = local write "Info："(w384) -> ()
                    n168 = local read "VCI_CAN_OBJ_T"() -> (w388:T2)
                    n169 = Bundle(cluster=w388, "ID"=w385, "TimeStamp"=u8 0 ("RemoteFlag"), "TimeFlag"=u8 1, "SendType"=u8 0 ("DataLen"), "RemoteFlag"=u8 0, "ExternFlag"=u8 1, "DataLen"=u8 8, u8 1 ("元素"), w395, w395, w395) -> (w392:T2)  [unwired: 7 in]
                    n170 = dll-call lib="PTH2{abs DPCTools2.sourceSNV-AutoTestV1.0.0ASettingsSEQEditDriver平台BCUAutoBurnSettingsControlCAN.dll" fn="VCI_Transmit"("DeviceType"=w391, "DeviceInd"=w390, "CANInd"=w389, "pSend"=w392, "Len"=u32 1) -> ()  [unwired: 5 in, 6 out]
                  }
                }
                n171 = local read "Info："() -> (w366:string)
                n172 = Concatenate Strings(w366, "boot就绪应答...成功" ("字符串"), "\n") -> (w369:string)
                n173 = local write "Info："(w369) -> ()
              }
            }
          }
          frame 233728..233760, 233983 {
            n174 = To Unsigned Byte Integer(number=w404) -> (unsigned 8bit integer=w403:u8)
            n175 = Equal?(x=w411, y=u8 85) -> (x = y?=w409:bool)
            n176 = case shown="False" w409 {
              tunnel: w408 -> [_ w442]
              tunnel: w407 -> [_ w441]
              tunnel: w406 -> [_ w440]
              tunnel: w405 -> [_ w439]
              tunnel: w403 -> [_ w436]
              frame False {
                n177 = local write "update flag"(FALSE ("update flag")) -> ()
                n178 = local read "Info："() -> (w414:string)
                n179 = Concatenate Strings(w414, "boot擦除flash应答...失败" ("字符串"), "\n") -> (w417:string)
                n180 = local write "Info："(w417) -> ()
                n181 = One Button Dialog(message="程序下载错误，请断电重试！" ("消息")) -> ()  [unwired: 1 in, 1 out]
                n182 = flat-sequence {
                  frame #0 {
                    n183 = local read "设备索引"() -> (w424:u32)
                    n184 = local read "CAN路数"() -> (w422:u32)
                    n185 = local read "波特率"() -> (w423:T1)
                    n186 = local read "滤波方式"() -> (w421:u8)
                    n187 = local read "工作方式"() -> (w420:u8)
                    n188 = local read "类型"() -> (w425:u32)
                    n189 = call "CAN_Init.vi"("设备类型"=w425, "设备索引"=w424, "波特率"=w423, "CAN路数"=w422, "操作类型"=enum16{"初始化CAN", "关闭CAN"}."关闭CAN", "滤波方式"=w421, "工作方式"=w420) -> ()  [unwired: 11 in, 2 out]
                    n190 = Wait (ms)(milliseconds to wait=u32 2000 ("等待时间（毫秒）")) -> ()  [unwired: 1 out]
                  }
                  frame #1 {
                    n191 = Quit LabVIEW(quit? (T)=TRUE ("退出？(T)")) -> ()
                  }
                }
              }
              frame True {
                w437 = 0 ("索引")
                n192 = local read "子数组"() -> (w438:string[])
                n193 = flat-sequence {
                  frame #0 {
                    n194 = local read "Info："() -> (w447:string)
                    n195 = Concatenate Strings(w447, "boot擦除flash应答...成功" ("字符串"), "\n") -> (w449:string)
                    n196 = local write "Info："(w449) -> ()
                  }
                  frame #1 {
                    n197 = local read "Info："() -> (w454:string)
                    n198 = Concatenate Strings(w454, "开始下载数据..." ("字符串"), "\n") -> (w452:string)
                    n199 = Tick Count (ms)() -> (millisecond timer value=w450:u32)
                    n200 = local write "Info："(w452) -> ()
                    n201 = local write "开始下载数据"(w450) -> ()
                    "开始下载数据" <- TRUE
                  }
                }
                n202 = Array Size(array=w438) -> (size(s)=w443:i32)
                n203 = Index Array(array=w438, index=w437) -> (element=w427:string)
                n204 = String Subset(string=w427, offset (0)=1 ("偏移量(0)"), length (rest)=1 ("长度（子字符串长度）")) -> (substring=w432:string)
                n205 = case shown="\"2\"" w432 {
                  tunnel: ["01" ("子字符串(\"\")") "02" ("子字符串(\"\")")] -> w431
                  frame "1", Default {
                  }
                  frame "2" {
                  }
                }
                n206 = String Subset(string=w427, offset (0)=2 ("偏移量(0)")) -> (substring=w429:string)  [unwired: 1 in]
                n207 = Concatenate Strings("FFFFFFFFFFFF" ("子字符串(\"\")"), w431, w429) -> ()  [unwired: 1 out]
                n208 = while {
                  tunnel: w442 -> [w479]
                  tunnel: w441 -> [w478]
                  tunnel: w440 -> [w477]
                  tunnel: w439 -> [w476]
                  shift-right: [w471] -> _
                  shift-left: w427 -> [w472]
                  tunnel: w443 -> [w469]
                  tunnel: w437 -> [w465]
                  tunnel: w436 -> [w459]
                  tunnel: u16 1 ("y") -> [w458]
                  stop <- w464 stop-if-true
                  w462 = u16 256 ("y")
                  n209 = String Length(string=w472) -> (length=w470:i32)
                  n210 = Greater Or Equal?(x=w470, y=16) -> (x >= y?=w473:bool)
                  n211 = local read "目标板类型"() -> (w457:enum16{"BCU/主板", "BMU/从板"})
                  n212 = case shown="\"BCU/主板\", Default" w457 {
                    tunnel: [u16 0 ("请选择板号") w481] -> w456
                    frame "BCU/主板", Default {
                    }
                    frame "BMU/从板" {
                      n213 = local read "请选择板号"() -> (w481:u16)
                    }
                  }
                  n214 = Multiply(x=w456, y=w462) -> ()  [unwired: 1 out]
                  n215 = Multiply(x=w462, y=w459) -> (x*y=w461:u16)
                  n216 = Divide(x=w465, y=w469) -> (x/y=w468:dbl)
                  n217 = Add(x=u32 262289 ("ID"), y=w461) -> (x+y=w460:u32)
                  n218 = Multiply(x=w468, y=100.0) -> (x*y=w466:dbl)
                  n219 = case shown="False" w473 {
                    tunnel: w479 -> [w510 w522]
                    tunnel: w478 -> [w509 w521]
                    tunnel: w477 -> [w508 w520]
                    tunnel: w476 -> [w507 w519]
                    tunnel: w472 -> [w483 w518]
                    tunnel: [w488 w517] -> w471
                    tunnel: [FALSE TRUE] -> w464
                    tunnel: w470 -> [_ w515]
                    tunnel: w470 -> [_ w514]
                    tunnel: w460 -> [w486 w513]
                    tunnel: w458 -> [_ w512]
                    frame True {
                      w504 = u8 0 ("元素")
                      n220 = String Subset(string=w483, length (rest)=16 ("长度（剩余）")) -> (substring=w482:string)  [unwired: 1 in]
                      n221 = String Subset(string=w483, offset (0)=16 ("偏移量(0)")) -> (substring=w488:string)  [unwired: 1 in]
                      n222 = call "ASCII_To_Hex.vi"("ASCII String"=w482) -> ("hex数组"=w484:u16[])  [unwired: 6 in, 4 out]
                      n223 = Index Array(array=w484) -> (element #1=w496:u16, element #2=w495:u16, element #3=w494:u16, element #4=w493:u16, element #5=w492:u16, element #6=w491:u16, element #7=w490:u16, element #8=w489:u16)  [unwired: 8 in]
                      n224 = Bundle(cluster=w510, "ID"=w486, "TimeStamp"=u8 0 ("RemoteFlag"), "TimeFlag"=u8 1, "SendType"=u8 0 ("DataLen"), "RemoteFlag"=u8 0, "ExternFlag"=u8 1, "DataLen"=u8 8, w496, w495, w494, w493, w492, w491, w490, w489, w504, w504, w504) -> (w499:T2)
                      n225 = dll-call lib="PTH2{abs DPCTools2.sourceSNV-AutoTestV1.0.0ASettingsSEQEditDriver平台BCUAutoBurnSettingsControlCAN.dll" fn="VCI_Transmit"("DeviceType"=w509, "DeviceInd"=w508, "CANInd"=w507, "pSend"=w499, "Len"=u32 1) -> ()  [unwired: 5 in, 6 out]
                    }
                    frame False {
                      n226 = Greater Than 0?(x=w515) -> (x > 0?=w511:bool)
                      n227 = case shown="True" w511 {
                        tunnel: w522 -> [w553 w563]
                        tunnel: w521 -> [w552 w562]
                        tunnel: w520 -> [w551 w561]
                        tunnel: w519 -> [w550 w560]
                        tunnel: w518 -> [w540 _]
                        tunnel: [w531 _] -> w517
                        tunnel: w514 -> [_ w558]
                        tunnel: w513 -> [w527 w557]
                        tunnel: w512 -> [_ w556]
                        tunnel: w512 -> [w526 _]
                        frame True {
                          w547 = u8 0 ("元素")
                          n228 = Wait (ms)(milliseconds to wait=u32 20 ("等待时间（毫秒）")) -> ()  [unwired: 1 out]
                          n229 = String Subset(string=w540, offset (0)=16 ("偏移量(0)")) -> (substring=w531:string)  [unwired: 1 in]
                          n230 = String Subset(string=w540, length (rest)=16 ("长度（剩余）")) -> (substring=w524:string)  [unwired: 1 in]
                          n231 = call "ASCII_To_Hex.vi"("ASCII String"=w524) -> ("hex数组"=w523:u16[])  [unwired: 6 in, 4 out]
                          n232 = Index Array(array=w523) -> (element #1=w539:u16, element #2=w538:u16, element #3=w537:u16, element #4=w536:u16, element #5=w535:u16, element #6=w534:u16, element #7=w533:u16, element #8=w532:u16)  [unwired: 8 in]
                          n233 = Bundle(cluster=w553, "ID"=w527, "TimeStamp"=u8 0 ("RemoteFlag"), "TimeFlag"=u8 1, "SendType"=u8 0 ("DataLen"), "RemoteFlag"=u8 0, "ExternFlag"=w526, "DataLen"=u8 8, w539, w538, w537, w536, w535, w534, w533, w532, w547, w547, w547) -> (w542:T2)
                          n234 = dll-call lib="PTH2{abs DPCTools2.sourceSNV-AutoTestV1.0.0ASettingsSEQEditDriver平台BCUAutoBurnSettingsControlCAN.dll" fn="VCI_Transmit"(error in="错误输入（无错误） 3", "DeviceType"=w552, "DeviceInd"=w551, "CANInd"=w550, "pSend"=w542, "Len"=u32 1) -> (error out=→"错误输出 14":errorcluster)  [unwired: 4 in, 5 out]
                        }
                        frame False {
                          (unwired) TRUE
                          n235 = Quotient & Remainder(x=w558, y=8) -> ()  [unwired: 2 out]
                          n236 = Wait (ms)(milliseconds to wait=u32 20 ("等待时间（毫秒）")) -> ()  [unwired: 1 out]
                          n237 = case shown="0" 1 {
                            tunnel: w563 -> [w588 _]
                            tunnel: w562 -> [w587 _]
                            tunnel: w561 -> [w586 _]
                            tunnel: w560 -> [w585 _]
                            tunnel: w557 -> [w565 _]
                            tunnel: w556 -> [w564 _]
                            frame 0 {
                              w582 = u8 0 ("元素")
                              n238 = Index Array(array=u8[] [0, 0, 0, 0, 0, 0, 0, 0] ("数组")) -> (element #1=w576:u8, element #2=w575:u8, element #3=w574:u8, element #4=w573:u8, element #5=w572:u8, element #6=w571:u8, element #7=w570:u8, element #8=w569:u8)  [unwired: 8 in]
                              n239 = Bundle(cluster=w588, "ID"=w565, "TimeStamp"=u8 0 ("RemoteFlag"), "TimeFlag"=u8 1, "SendType"=u8 0 ("DataLen"), "RemoteFlag"=u8 0, "ExternFlag"=w564, "DataLen"=u8 8, w576, w575, w574, w573, w572, w571, w570, w569, w582, w582, w582) -> (w577:T2)
                              n240 = dll-call lib="PTH2{abs DPCTools2.sourceSNV-AutoTestV1.0.0ASettingsSEQEditDriver平台BCUAutoBurnSettingsControlCAN.dll" fn="VCI_Transmit"(error in="错误输入（无错误） 4", "DeviceType"=w587, "DeviceInd"=w586, "CANInd"=w585, "pSend"=w577, "Len"=u32 1) -> (error out=→"错误输出 15":errorcluster)  [unwired: 4 in, 5 out]
                            }
                            frame 1, Default {
                            }
                          }
                        }
                      }
                    }
                  }
                  n241 = local write "进度"(w466) -> ()
                  n242 = Wait (ms)(milliseconds to wait=u32 5 ("等待时间（毫秒）")) -> ()  [unwired: 1 out]
                }
                "当前发送行" <- w437
              }
            }
          }
          frame 299264..299296, 299519 {
            n243 = To Unsigned Byte Integer(number=w592) -> (unsigned 8bit integer=w591:u8)
            n244 = Equal?(x=w590, y=u8 85) -> (x = y?=w589:bool)
            n245 = case shown="False" w589 {
              tunnel: w596 -> [_ w622]
              tunnel: w595 -> [_ w621]
              tunnel: w594 -> [_ w620]
              tunnel: w593 -> [_ w619]
              tunnel: w591 -> [_ w613]
              frame False {
                n246 = local write "update flag"(FALSE ("update flag")) -> ()
                n247 = local read "Info："() -> (w600:string)
                n248 = Concatenate Strings(w600, "扇区数据传输应答...失败" ("字符串"), "\n") -> (w603:string)
                n249 = One Button Dialog(message="程序下载错误，请断电重试！" ("消息")) -> ()  [unwired: 1 in, 1 out]
                n250 = local write "Info："(w603) -> ()
              }
              frame True {
                n251 = local read "当前发送行"() -> (w617:i32)
                n252 = local read "子数组"() -> (w618:string[])
                n253 = Array Size(array=w618) -> (size(s)=w623:i32)
                n254 = Increment(x=w617) -> (x+1=w616:i32)
                n255 = Index Array(array=w618, index=w616) -> (element=w605:string)
                n256 = String Subset(string=w605, offset (0)=1 ("偏移量(0)"), length (rest)=1 ("长度（子字符串长度）")) -> (substring=w610:string)
                n257 = case shown="\"2\"" w610 {
                  tunnel: ["01" ("子字符串(\"\")") "02" ("子字符串(\"\")")] -> w608
                  frame "1", Default {
                  }
                  frame "2" {
                  }
                }
                n258 = Tick Count (ms)() -> (millisecond timer value=w604:u32)
                n259 = local write "当前发送行"(w616) -> ()
                n260 = String Subset(string=w605, offset (0)=2 ("偏移量(0)")) -> (substring=w606:string)  [unwired: 1 in]
                n261 = String Length(string=w605) -> (length=w615:i32)
                n262 = local write "开始下载数据"(w604) -> ()
                n263 = Concatenate Strings("FFFFFFFFFFFF" ("子字符串(\"\")"), w608, w606) -> ()  [unwired: 1 out]
                n264 = Greater Than 0?(x=w615) -> (x > 0?=w614:bool)
                n265 = case shown="False" w614 {
                  tunnel: w623 -> [_ w688]
                  tunnel: w622 -> [w667 w687]
                  tunnel: w621 -> [w666 w686]
                  tunnel: w620 -> [w665 w685]
                  tunnel: w619 -> [w664 w684]
                  tunnel: w616 -> [_ w683]
                  tunnel: w605 -> [_ w682]
                  tunnel: w613 -> [w637 w677]
                  frame False {
                    w628 = "BURNRESULT" ("section")
                    w661 = u8 0 ("元素")
                    n266 = Multiply(x=w637, y=u16 256) -> (x*y=w634:u16)
                    n267 = local write "update flag"(FALSE ("update flag")) -> ()
                    n268 = local write "开始下载数据"(FALSE ("开始下载数据")) -> ()
                    n269 = Add(x=u32 327825 ("ID"), y=w634) -> (x+y=w635:u32)
                    n270 = String To Byte Array(string="" ("字符串")) -> (unsigned byte array=w655:u8[])
                    n271 = flat-sequence {
                      frame #0 {
                        n272 = local read "设备索引"() -> (w674:u32)
                        n273 = local read "CAN路数"() -> (w672:u32)
                        n274 = local read "波特率"() -> (w673:T1)
                        n275 = local read "滤波方式"() -> (w671:u8)
                        n276 = local read "工作方式"() -> (w670:u8)
                        n277 = local read "类型"() -> (w675:u32)
                        n278 = call "CAN_Init.vi"("设备类型"=w675, "设备索引"=w674, "波特率"=w673, "CAN路数"=w672, "操作类型"=enum16{"初始化CAN", "关闭CAN"}."关闭CAN", "滤波方式"=w671, "工作方式"=w670) -> ()  [unwired: 11 in, 2 out]
                        n279 = Wait (ms)(milliseconds to wait=u32 2000 ("等待时间（毫秒）")) -> ()  [unwired: 1 out]
                      }
                      frame #1 {
                        n280 = Quit LabVIEW(quit? (T)=TRUE ("退出？(T)")) -> ()
                      }
                    }
                    n281 = Index Array(array=w655) -> (element #1=w654:u8, element #2=w653:u8, element #3=w652:u8, element #4=w651:u8, element #5=w650:u8, element #6=w649:u8, element #7=w648:u8, element #8=w647:u8)  [unwired: 8 in]
                    n282 = Bundle(cluster=w667, "ID"=w635, "TimeStamp"=u8 0 ("RemoteFlag"), "TimeFlag"=u8 1, "SendType"=u8 0 ("DataLen"), "RemoteFlag"=u8 0, "ExternFlag"=u8 1, "DataLen"=u8 8, w654, w653, w652, w651, w650, w649, w648, w647, w661, w661, w661) -> (w656:T2)
                    n283 = dll-call lib="PTH2{abs DPCTools2.sourceSNV-AutoTestV1.0.0ASettingsSEQEditDriver平台BCUAutoBurnSettingsControlCAN.dll" fn="VCI_Transmit"(error in="错误输入（无错误） 7", "DeviceType"=w666, "DeviceInd"=w665, "CANInd"=w664, "pSend"=w656, "Len"=u32 1) -> (error out=→"错误输出 18":errorcluster)  [unwired: 4 in, 5 out]
                    n284 = local read "Info："() -> (w640:string)
                    n285 = call <vilib>:"Open Config Data.vi"("configuration file path"=path "D:/BlueWay/configresult.ini") -> ("refnum"=w627:T4)  [unwired: 8 in, 2 out]
                    n286 = Concatenate Strings(w640, "应用刷写完成..请重新上电！" ("字符串"), "\n") -> (w643:string)
                    n287 = local write "Info："(w643) -> ()
                    n288 = call-poly <vilib>:"Write Key.vi"("section"=w628, "value"="PASS" ("section"), "key"=w628, "refnum"=w627) -> ("error out"=w631:errorcluster, "refnum out"=w630:T4)  [unwired: 5 in, 1 out]
                    n289 = call <vilib>:"Close Config Data.vi"("error in (no error)"=w631, "refnum"=w630) -> ()  [unwired: 8 in, 2 out]
                  }
                  frame True {
                    n290 = Multiply(x=w677, y=u16 256) -> (x*y=w680:u16)
                    n291 = Add(x=u32 262289 ("ID"), y=w680) -> (x+y=w678:u32)
                    n292 = while {
                      tunnel: w687 -> [w704]
                      tunnel: w686 -> [w703]
                      tunnel: w685 -> [w702]
                      tunnel: w684 -> [w701]
                      shift-right: [w697] -> _
                      shift-left: w682 -> [w698]
                      tunnel: w688 -> [w695]
                      tunnel: w683 -> [w691]
                      tunnel: w678 -> [w689]
                      stop <- w690 stop-if-true
                      n293 = String Length(string=w698) -> (length=w696:i32)
                      n294 = Greater Or Equal?(x=w696, y=16) -> (x >= y?=w699:bool)
                      n295 = case shown="True" w699 {
                        tunnel: w704 -> [w733 w745]
                        tunnel: w703 -> [w732 w744]
                        tunnel: w702 -> [w731 w743]
                        tunnel: w701 -> [w730 w742]
                        tunnel: w698 -> [w720 w741]
                        tunnel: [w710 w740] -> w697
                        tunnel: [FALSE TRUE] -> w690
                        tunnel: w696 -> [_ w738]
                        tunnel: w696 -> [_ w737]
                        tunnel: w689 -> [w708 w735]
                        frame True {
                          (unwired) u8 1 ("ExternFlag")
                          w727 = u8 0 ("元素")
                          n296 = String Subset(string=w720, offset (0)=16 ("偏移量(0)")) -> (substring=w710:string)  [unwired: 1 in]
                          n297 = String Subset(string=w720, length (rest)=16 ("长度（剩余）")) -> (substring=w706:string)  [unwired: 1 in]
                          n298 = call "ASCII_To_Hex.vi"("ASCII String"=w706) -> ("hex数组"=w705:u16[])  [unwired: 6 in, 4 out]
                          n299 = Index Array(array=w705) -> (element #1=w718:u16, element #2=w717:u16, element #3=w716:u16, element #4=w715:u16, element #5=w714:u16, element #6=w713:u16, element #7=w712:u16, element #8=w711:u16)  [unwired: 8 in]
                          n300 = Bundle(cluster=w733, "ID"=w708, "TimeStamp"=u8 0 ("RemoteFlag"), "TimeFlag"=u8 1, "SendType"=u8 0 ("DataLen"), "RemoteFlag"=u8 0, "ExternFlag"=u8 1, "DataLen"=u8 8, w718, w717, w716, w715, w714, w713, w712, w711, w727, w727, w727) -> (w722:T2)
                          n301 = dll-call lib="PTH2{abs DPCTools2.sourceSNV-AutoTestV1.0.0ASettingsSEQEditDriver平台BCUAutoBurnSettingsControlCAN.dll" fn="VCI_Transmit"("DeviceType"=w732, "DeviceInd"=w731, "CANInd"=w730, "pSend"=w722, "Len"=u32 1) -> ()  [unwired: 5 in, 6 out]
                        }
                        frame False {
                          n302 = Greater Than 0?(x=w738) -> ()  [unwired: 1 out]
                          n303 = case shown="True" TRUE {
                            tunnel: w745 -> [w776 w783]
                            tunnel: w744 -> [w775 w782]
                            tunnel: w743 -> [w774 w781]
                            tunnel: w742 -> [w773 w780]
                            tunnel: w741 -> [w763 _]
                            tunnel: [w754 _] -> w740
                            tunnel: w737 -> [_ w778]
                            tunnel: w735 -> [w751 _]
                            tunnel: [w749 _] -> w734
                            frame True {
                              w770 = u8 0 ("元素")
                              n304 = String Subset(string=w763, length (rest)=16 ("长度（剩余）")) -> (substring=w748:string)  [unwired: 1 in]
                              n305 = String Subset(string=w763, offset (0)=16 ("偏移量(0)")) -> (substring=w754:string)  [unwired: 1 in]
                              n306 = call "ASCII_To_Hex.vi"("ASCII String"=w748) -> ("hex数组"=w747:u16[])  [unwired: 6 in, 4 out]
                              n307 = Index Array(array=w747) -> (element #1=w762:u16, element #2=w761:u16, element #3=w760:u16, element #4=w759:u16, element #5=w758:u16, element #6=w757:u16, element #7=w756:u16, element #8=w755:u16)  [unwired: 8 in]
                              n308 = Bundle(cluster=w776, "ID"=w751, "TimeStamp"=u8 0 ("RemoteFlag"), "TimeFlag"=u8 1, "SendType"=u8 0 ("DataLen"), "RemoteFlag"=u8 0, "ExternFlag"=u8 1, "DataLen"=u8 8, w762, w761, w760, w759, w758, w757, w756, w755, w770, w770, w770) -> (w765:T2)
                              n309 = dll-call lib="PTH2{abs DPCTools2.sourceSNV-AutoTestV1.0.0ASettingsSEQEditDriver平台BCUAutoBurnSettingsControlCAN.dll" fn="VCI_Transmit"(error in="错误输入（无错误） 5", "DeviceType"=w775, "DeviceInd"=w774, "CANInd"=w773, "pSend"=w765, "Len"=u32 1) -> (error out=w749:errorcluster)  [unwired: 4 in, 5 out]
                              "错误输出 16" <- w749
                            }
                            frame False {
                              n310 = Quotient & Remainder(x=w778, y=8) -> (x-y*floor(x/y)=w777:i32)  [unwired: 1 out]
                              n311 = case shown="0" w777 {
                                tunnel: w783 -> [w807 _]
                                tunnel: w782 -> [w806 _]
                                tunnel: w781 -> [w805 _]
                                tunnel: w780 -> [w804 _]
                                frame 0 {
                                w800 = u8 0 ("元素")
                                n312 = Index Array(array=u8[] [0, 0, 0, 0, 0, 0, 0, 0] ("数组")) -> (element #1=w794:u8, element #2=w793:u8, element #3=w792:u8, element #4=w791:u8, element #5=w790:u8, element #6=w789:u8, element #7=w788:u8, element #8=w787:u8)  [unwired: 8 in]
                                n313 = Bundle(cluster=w807, "ID"=u32 5, "TimeStamp"=u8 0 ("RemoteFlag"), "TimeFlag"=u8 1, "SendType"=u8 0 ("DataLen"), "RemoteFlag"=u8 0, "DataLen"=u8 8, w794, w793, w792, w791, w790, w789, w788, w787, w800, w800, w800) -> (w795:T2)  [unwired: 1 in]
                                n314 = dll-call lib="PTH2{abs DPCTools2.sourceSNV-AutoTestV1.0.0ASettingsSEQEditDriver平台BCUAutoBurnSettingsControlCAN.dll" fn="VCI_Transmit"(error in="错误输入（无错误） 6", "DeviceType"=w806, "DeviceInd"=w805, "CANInd"=w804, "pSend"=w795, "Len"=u32 1) -> (error out=→"错误输出 17":errorcluster)  [unwired: 4 in, 5 out]
                                }
                                frame 1, Default {
                                }
                              }
                            }
                          }
                          n315 = flat-sequence {
                            tunnel: w734 -> [_]
                            frame #0 {
                              n316 = Wait (ms)(milliseconds to wait=u32 1 ("等待时间（毫秒）")) -> ()  [unwired: 1 out]
                            }
                          }
                        }
                      }
                      n317 = Divide(x=w691, y=w695) -> (x/y=w694:dbl)
                      n318 = Multiply(x=w694, y=100.0) -> (x*y=w692:dbl)
                      n319 = local write "进度"(w692) -> ()
                    }
                  }
                }
              }
            }
          }
          frame 254 {
            (unwired) TRUE
            n320 = disable-structure shown="禁用" {
              disable-tunnel: w814 -> [w824 _]
              disable-tunnel: w813 -> [w823 _]
              disable-tunnel: w812 -> [w822 _]
              disable-tunnel: w811 -> [w821 _]
              disable-tunnel: w808 -> [w817 _]
              frame Disabled {
                w820 = FALSE ("进入烧录模式")
                n321 = Two Button Dialog(message="进入烧录模式!，是否开始烧录？\n如果BMS重新上电，请点取消！！" ("消息")) -> (T button?=w815:bool)  [unwired: 2 in]
                n322 = case shown="True" w815 {
                  tunnel: w824 -> [w830 w857]
                  tunnel: w823 -> [w829 w852]
                  tunnel: w822 -> [w828 w851]
                  tunnel: w821 -> [w827 w850]
                  tunnel: w817 -> [w825 w853]
                  frame True {
                    n323 = stacked-sequence {
                      tunnel: w830 -> [_ w838]
                      tunnel: w829 -> [w833 w837]
                      tunnel: w828 -> [w832 w836]
                      tunnel: w827 -> [w831 w835]
                      tunnel: w825 -> [w834 _]
                      frame #0 {
                        n324 = Flush Queue(queue=w834) -> ()  [unwired: 1 in, 3 out]
                        n325 = dll-call lib="PTH2{abs DPCTools2.sourceSNV-AutoTestV1.0.0ASettingsSEQEditDriver平台BCUAutoBurnSettingsControlCAN.dll" fn="VCI_ClearBuffer" label="VCI_Clearbuffer"("DeviceType"=w833, "DeviceInd"=w832, "CANInd"=w831) -> ()  [unwired: 4 in, 5 out]
                      }
                      frame #1 {
                        w845 = u8 0 ("元素")
                        n326 = Bundle(cluster=w838, "ID"=u32 0, "TimeStamp"=u8 0 ("RemoteFlag"), "TimeFlag"=u8 1, "SendType"=u8 0 ("DataLen"), "RemoteFlag"=u8 0, "ExternFlag"=u8 0, "DataLen"=u8 1, u8 2 ("元素"), w845, w845, w845) -> (w849:T2)  [unwired: 7 in]
                        n327 = dll-call lib="PTH2{abs DPCTools2.sourceSNV-AutoTestV1.0.0ASettingsSEQEditDriver平台BCUAutoBurnSettingsControlCAN.dll" fn="VCI_Transmit"("DeviceType"=w837, "DeviceInd"=w836, "CANInd"=w835, "pSend"=w849, "Len"=u32 1) -> ()  [unwired: 5 in, 6 out]
                      }
                    }
                    "进入烧录模式" <- TRUE ("进入烧录模式")
                  }
                  frame False {
                    n328 = Flush Queue(queue=w853) -> (error out=w855:errorcluster)  [unwired: 1 in, 2 out]
                    n329 = invoke on="Monitor" class="Bool" method="Reinit To Default"() -> ()  [unwired: 3 in, 3 out]
                    n330 = local write "Monitor_flag"(FALSE ("Monitor_flag")) -> ()
                    n331 = dll-call lib="PTH2{abs DPCTools2.sourceSNV-AutoTestV1.0.0ASettingsSEQEditDriver平台BCUAutoBurnSettingsControlCAN.dll" fn="VCI_ClearBuffer" label="VCI_Clearbuffer"(error in=w855, "DeviceType"=w852, "DeviceInd"=w851, "CANInd"=w850) -> (error out=w854:errorcluster)  [unwired: 3 in, 4 out]
                    n332 = disable-structure shown="禁用" {
                      disable-tunnel: w857 -> [w862 _]
                      disable-tunnel: w854 -> [w861 _]
                      disable-tunnel: w852 -> [w860 _]
                      disable-tunnel: w851 -> [w859 _]
                      disable-tunnel: w850 -> [w858 _]
                      frame Disabled {
                        w869 = u8 0 ("元素")
                        n333 = Bundle(cluster=w862, "ID"=u32 0, "TimeStamp"=u8 0 ("RemoteFlag"), "TimeFlag"=u8 1, "SendType"=u8 0 ("DataLen"), "RemoteFlag"=u8 0, "ExternFlag"=u8 0, "DataLen"=u8 1, u8 5 ("元素"), w869, w869, w869) -> (w873:T2)  [unwired: 7 in]
                        n334 = dll-call lib="PTH2{abs DPCTools2.sourceSNV-AutoTestV1.0.0ASettingsSEQEditDriver平台BCUAutoBurnSettingsControlCAN.dll" fn="VCI_Transmit"(error in=w861, "DeviceType"=w860, "DeviceInd"=w859, "CANInd"=w858, "pSend"=w873, "Len"=u32 1) -> ()  [unwired: 4 in, 6 out]
                      }
                      frame Enabled {
                      }
                    }
                  }
                }
                n335 = property on="烧录结果" class="Bool (strict)"("Colors [4]"=cluster{u32, u32}[] [{0, 0}] ("颜色[4]"), "BoolText.Text"="" ("布尔文本.文本")) -> ()  [unwired: 2 in, 2 out]
                n336 = local write "擦除完成"(w820) -> ()
                n337 = local write "烧录结果"(w820) -> ()
              }
              frame Enabled {
              }
            }
          }
          frame 253 {
            n338 = disable-structure shown="禁用" {
              disable-tunnel: w883 -> [w893 _]
              disable-tunnel: [w892 _] -> w882
              disable-tunnel: w881 -> [w891 _]
              disable-tunnel: w880 -> [w890 _]
              disable-tunnel: w879 -> [w889 _]
              disable-tunnel: w878 -> [w888 _]
              disable-tunnel: w877 -> [w887 _]
              disable-tunnel: [w886 _] -> w876
              disable-tunnel: w875 -> [w885 _]
              disable-tunnel: w874 -> [w884 _]
              frame Disabled {
                n339 = stacked-sequence {
                  tunnel: w893 -> [_ w911]
                  tunnel: [_ w910] -> w892
                  tunnel: w891 -> [w898 w909]
                  tunnel: w890 -> [w897 w908]
                  tunnel: w889 -> [_ w907]
                  tunnel: w888 -> [w896 w906]
                  tunnel: w887 -> [_ w905]
                  tunnel: [_ w904] -> w886
                  tunnel: w885 -> [_ w903]
                  tunnel: w884 -> [w895 w899]
                  frame #0 {
                    n340 = dll-call lib="PTH2{abs DPCTools2.sourceSNV-AutoTestV1.0.0ASettingsSEQEditDriver平台BCUAutoBurnSettingsControlCAN.dll" fn="VCI_ClearBuffer" label="VCI_Clearbuffer"("DeviceType"=w898, "DeviceInd"=w897, "CANInd"=w896) -> ()  [unwired: 4 in, 5 out]
                    n341 = Flush Queue(queue=w895) -> ()  [unwired: 1 in, 3 out]
                  }
                  frame #1 {
                    # "FD"
                    n342 = local read "子数组"() -> (w913:string[])
                    n343 = while {
                      tunnel: w913 -> [w984] mode=indexing
                      tunnel: [w980] -> w912
                      tunnel: [w976] -> w902
                      i -> [w980]
                      stop <- w977 stop-if-true
                      n344 = Search/Split String(string=w984, search string/char (-)="S9" ("搜索字符串/字符(-)")) -> (offset of match=w982:i32)  [unwired: 1 in, 2 out]
                      n345 = Equal?(x=5000, y=w980) -> (x = y?=w978:bool)
                      n346 = Not Equal?(x=w982, y=-1) -> (x != y?=w976:bool)
                      n347 = Or(x=w976, y=w978) -> (x .or. y?=w977:bool)
                    }
                    n348 = while {
                      tunnel: w913 -> [w993] mode=indexing
                      tunnel: [w986] -> w900
                      tunnel: [w985] -> w901
                      i -> [w986]
                      stop <- w988 stop-if-true
                      n349 = Equal?(x=5000, y=w986) -> (x = y?=w987:bool)
                      n350 = Search/Split String(string=w993, search string/char (-)="S0" ("搜索字符串/字符(-)")) -> (offset of match=w991:i32)  [unwired: 1 in, 2 out]
                      n351 = Not Equal?(x=w991, y=-1) -> (x != y?=w985:bool)
                      n352 = Or(x=w985, y=w987) -> (x .or. y?=w988:bool)
                    }
                    n353 = case shown="True" w902 {
                      tunnel: w913 -> [_ w959]
                      tunnel: w912 -> [_ w958]
                      tunnel: w911 -> [w915 _]
                      tunnel: [w915 w925] -> w910
                      tunnel: w909 -> [_ w957]
                      tunnel: w908 -> [_ w956]
                      tunnel: w907 -> [_ _]
                      tunnel: w906 -> [_ w955]
                      tunnel: w905 -> [w914 w940]
                      tunnel: [w914 w938] -> w904
                      tunnel: w903 -> [_ w922]
                      tunnel: w901 -> [_ w921]
                      tunnel: w900 -> [_ w920]
                      tunnel: w899 -> [_ w916]
                      frame False {
                      }
                      frame True {
                        n354 = case shown="True" w921 {
                          tunnel: w920 -> [_ w962]
                          tunnel: [0 w963] -> w919
                          tunnel: [-1 w962] -> w918
                          frame False {
                          }
                          frame True {
                            n355 = Increment(x=w962) -> (x+1=w963:i32)
                          }
                        }
                        n356 = Subtract(x=w958, y=w918) -> (x-y=w932:i32)
                        n357 = Decrement(x=w932) -> (x-1=w931:i32)
                        n358 = Array Subset(array=w959, index=w919, length=w931) -> (w929:string[])
                        n359 = Index Array(array=w929, index=0 ("索引")) -> (element=w937:string)
                        n360 = Delete From Array(array=w929, length=1 ("长度"), index=0 ("索引")) -> (array with subset deleted=w925:string[])  [unwired: 1 out]
                        n361 = String Subset(string=w937, offset (0)=0 ("偏移量(0)"), length (rest)=2 ("长度（剩余）")) -> (substring=w947:string)
                        n362 = String Subset(string=w937, offset (0)=2 ("偏移量(0)"), length (rest)=2 ("长度（剩余）")) -> (substring=w950:string)
                        n363 = Hexadecimal String To Number(string=w950) -> (number=w945:u32)  [unwired: 2 in, 1 out]
                        n364 = case shown="\"S2\"" w947 {
                          tunnel: [4 ("偏移量(0)") 6 ("偏移量(0)")] -> w936
                          tunnel: w945 -> [w968 w974]
                          tunnel: [w966 w972] -> w944
                          tunnel: [8 ("y") 10 ("y")] -> w941
                          tunnel: ["S1" "S2"] -> w933
                          frame "S1", Default {
                            n365 = Subtract(x=w968, y=3) -> (x-y=w966:u32)
                          }
                          frame "S2" {
                            n366 = Subtract(x=w974, y=4) -> (x-y=w972:u32)
                          }
                        }
                        "地址长度" <- w936
                        n367 = Array Size(array=w925) -> (size(s)=w926:i32)
                        "大小" <- w926
                        n368 = Divide(x=0, y=w926) -> (x/y=w923:dbl)
                        n369 = local write "进度"(w923) -> ()
                        n370 = String Subset(string=w937, offset (0)=4 ("偏移量(0)"), length (rest)=w936) -> ()  [unwired: 1 out]
                        n371 = Multiply(x=u32 2, y=w944) -> (x*y=w942:u32)
                        "数据长度" <- w942
                        n372 = String Subset(string=w937, offset (0)=4 ("偏移量(0)"), length (rest)=w936) -> (substring=w934:string)
                        n373 = call "CAN R&W.vi"("设备类型"=w957, "设备索引"=w956, "CAN路数"=w955, "DataLen"=u8 8, "写地址/数据"=enum16{"写地址", "写数据"}."写地址", "Data Input"=w934, "枚举"=w922, "TYPE"=w933, "queue out"=w916) -> ("发送的数据"=→"发送的数据":i32[])  [unwired: 17 in, 1 out]
                        n374 = String Subset(string=w937, offset (0)=w941, length (rest)=w942) -> (substring=w939:string)
                        n375 = Concatenate Strings(w940, w939) -> (w938:string)
                      }
                    }
                  }
                }
                "擦除完成" <- TRUE ("擦写状态")
              }
              frame Enabled {
              }
            }
          }
          frame 252 {
            n376 = Unbundle(w995) -> (w996:u8, w997:u8, w998:u8, w999:u8, w1000:u8, w1001:u8, w1002:u8, w1003:u8)  [unwired: 10 out]
            n377 = Build Array(w996, w997, w998, w999, w1000, w1001, w1002, w1003) -> (w994:u8[])
            n378 = disable-structure shown="禁用" {
              disable-tunnel: w1011 -> [w1020 _]
              disable-tunnel: [w1019 _] -> w1010
              disable-tunnel: w1009 -> [w1018 _]
              disable-tunnel: w1008 -> [w1017 _]
              disable-tunnel: w1007 -> [w1016 _]
              disable-tunnel: w1006 -> [w1015 _]
              disable-tunnel: w1005 -> [w1014 _]
              disable-tunnel: w1004 -> [w1013 _]
              disable-tunnel: w994 -> [w1012 _]
              frame Disabled {
                n379 = stacked-sequence {
                  tunnel: w1020 -> [_ w1043]
                  tunnel: [_ w1042] -> w1019
                  tunnel: w1018 -> [w1024 w1041]
                  tunnel: w1017 -> [w1023 w1040]
                  tunnel: w1016 -> [w1022 w1039]
                  tunnel: w1015 -> [_ w1037]
                  tunnel: w1014 -> [_ w1036]
                  tunnel: w1012 -> [_ w1030]
                  tunnel: w1013 -> [w1021 w1025]
                  frame #0 {
                    n380 = dll-call lib="PTH2{abs DPCTools2.sourceSNV-AutoTestV1.0.0ASettingsSEQEditDriver平台BCUAutoBurnSettingsControlCAN.dll" fn="VCI_ClearBuffer" label="VCI_Clearbuffer"("DeviceType"=w1024, "DeviceInd"=w1023, "CANInd"=w1022) -> ()  [unwired: 4 in, 5 out]
                    n381 = Flush Queue(queue=w1021) -> ()  [unwired: 1 in, 3 out]
                  }
                  frame #1 {
                    # "FC"
                    n382 = local read "发送的数据"() -> (w1035:i32[])
                    n383 = String Length(string=w1043) -> (length=w1044:i32)
                    n384 = Array Subset(array=w1030, index=1 ("索引"), length=6 ("长度")) -> (w1028:u8[])
                    n385 = Array Size(array=w1037) -> (size(s)=w1038:i32)
                    n386 = Array Subset(array=w1035, index=1 ("索引"), length=6 ("长度")) -> (w1029:i32[])
                    n387 = Greater Than 0?(x=w1044) -> (x > 0?=w1045:bool)
                    n388 = Equal?(x=w1029, y=w1028) -> (x = y?=w1027:bool[])
                    n389 = And Array Elements(Boolean array=w1027) -> (logical AND=w1026:bool)
                    n390 = case shown="False" w1026 {
                      tunnel: w1045 -> [_ w1057]
                      tunnel: w1044 -> [_ w1056]
                      tunnel: w1043 -> [_ w1055]
                      tunnel: [_ w1054] -> w1042
                      tunnel: w1041 -> [_ w1053]
                      tunnel: w1040 -> [_ w1052]
                      tunnel: w1039 -> [_ w1051]
                      tunnel: w1038 -> [_ w1050]
                      tunnel: w1036 -> [_ w1049]
                      tunnel: w1025 -> [_ w1048]
                      frame False {
                        w1046 = "失败" ("布尔文本.文本")
                        w1047 = cluster{u32, u32}[] [{16711680, 0}] ("颜色[4]")
                        n391 = property on="校验" class="Bool (strict)"("Colors [4]"=w1047, "BoolText.Text"=w1046) -> ()  [unwired: 2 in, 2 out]
                        n392 = property on="烧录结果" class="Bool (strict)"("Colors [4]"=w1047, "BoolText.Text"=w1046) -> ()  [unwired: 2 in, 2 out]
                      }
                      frame True {
                        n393 = case shown="False" w1057 {
                          tunnel: w1056 -> [_ w1071]
                          tunnel: w1055 -> [w1058 w1072]
                          tunnel: [w1058 w1070] -> w1054
                          tunnel: w1053 -> [_ w1067]
                          tunnel: w1052 -> [_ w1066]
                          tunnel: w1051 -> [_ w1065]
                          tunnel: w1050 -> [_ _]
                          tunnel: w1049 -> [_ w1061]
                          tunnel: w1048 -> [_ w1059]
                          frame False {
                          }
                          frame True {
                            n394 = Quotient & Remainder(x=w1071, y=12) -> (x-y*floor(x/y)=w1063:i32, floor(x/y)=w1062:i32)
                            n395 = Greater Than 0?(x=w1062) -> (x > 0?=w1073:bool)
                            n396 = case shown="True" w1073 {
                              tunnel: w1072 -> [w1089 w1112]
                              tunnel: w1071 -> [_ w1109]
                              tunnel: ["" w1108] -> w1070
                              tunnel: [w1076 w1107] -> w1068
                              tunnel: w1063 -> [w1086 _]
                              tunnel: [w1077 u8 8 ("DataLen")] -> w1064
                              tunnel: w1061 -> [w1075 _]
                              frame False {
                                n397 = Divide(x=w1086, y=2) -> (x/y=w1081:dbl)
                                "发送数据长度" <- w1081
                                n398 = String Subset(string=w1089, length (rest)=w1086) -> (substring=w1079:string)  [unwired: 1 in]
                                n399 = Increment(x=w1081) -> (x+1=w1085:dbl)
                                n400 = Increment(x=w1085) -> (x+1=w1078:dbl)
                                n401 = Quotient & Remainder(x=w1081, y=2.0) -> (x-y*floor(x/y)=w1083:dbl)  [unwired: 1 out]
                                n402 = Equal?(x=w1083, y=1.0) -> (x = y?=w1080:bool)
                                n403 = case shown="True" w1080 {
                                tunnel: w1079 -> [w1090 w1094]
                                tunnel: w1078 -> [w1091 w1096]
                                tunnel: [w1091 w1095] -> w1077
                                tunnel: [w1090 w1093] -> w1076
                                tunnel: w1075 -> [_ w1092]
                                frame False {
                                }
                                frame True {
                                n404 = case shown="\"主板\"" w1092 {
                                tunnel: w1096 -> [w1100 w1103]
                                tunnel: [w1099 w1103] -> w1095
                                tunnel: w1094 -> [w1098 w1102]
                                tunnel: [w1097 w1102] -> w1093
                                frame "主板" {
                                n405 = Concatenate Strings(w1098, "FF") -> (w1097:string)
                                n406 = Increment(x=w1100) -> (x+1=w1099:dbl)
                                }
                                frame "从板", Default {
                                }
                                }
                                }
                                }
                              }
                              frame True {
                                w1106 = 12 ("长度（剩余）")
                                n407 = Subtract(x=w1109, y=12 ("长度（剩余）")) -> (x-y=w1111:i32)
                                n408 = String Subset(string=w1112, offset (0)=w1106, length (rest)=w1111) -> (substring=w1108:string)
                                n409 = String Subset(string=w1112, length (rest)=w1106) -> (substring=w1107:string)  [unwired: 1 in]
                                n410 = local write "发送数据长度"(6.0 ("发送数据长度")) -> ()
                              }
                            }
                            n411 = call "CAN R&W.vi"("设备类型"=w1067, "设备索引"=w1066, "CAN路数"=w1065, "DataLen"=w1064, "写地址/数据"=enum16{"写地址", "写数据"}."写数据", "Data Input"=w1068, "枚举"=w1061, "queue out"=w1059) -> ("发送的数据"=w1060:i32[])  [unwired: 18 in, 1 out]
                            n412 = local write "发送的数据"(w1060) -> ()
                          }
                        }
                      }
                    }
                  }
                }
              }
              frame Enabled {
              }
            }
          }
          frame 251 {
            n413 = disable-structure shown="禁用" {
              disable-tunnel: w1123 -> [w1152 _]
              disable-tunnel: w1122 -> [w1151 _]
              disable-tunnel: w1121 -> [w1150 _]
              disable-tunnel: [w1148 _] -> w1120
              disable-tunnel: w1119 -> [w1147 _]
              disable-tunnel: [w1145 _] -> w1118
              disable-tunnel: w1117 -> [w1144 _]
              disable-tunnel: w1116 -> [w1143 _]
              disable-tunnel: w1115 -> [w1142 _]
              disable-tunnel: w1114 -> [w1134 _]
              disable-tunnel: w1113 -> [w1125 _]
              frame Disabled {
                w1139 = 1 ("索引")
                # "FB"
                n414 = Unbundle(w1125) -> (w1126:u8, w1127:u8, w1128:u8, w1129:u8, w1130:u8, w1131:u8, w1132:u8, w1133:u8)  [unwired: 10 out]
                n415 = Build Array(w1126, w1127, w1128, w1129, w1130, w1131, w1132, w1133) -> (w1124:u8[])
                n416 = local read "发送数据长度"() -> (w1140:dbl)
                n417 = local read "发送的数据"() -> (w1141:i32[])
                n418 = String Length(string=w1147) -> (length=w1149:i32)
                n419 = Array Subset(array=w1141, index=w1139, length=w1140) -> (w1137:i32[])
                n420 = Array Subset(array=w1124, index=w1139, length=w1139) -> (w1136:u8[])
                n421 = Array Size(array=w1144) -> (size(s)=w1146:i32)
                n422 = Greater Than 0?(x=w1149) -> (x > 0?=w1153:bool)
                n423 = Equal?(x=w1137, y=w1136) -> (x = y?=w1138:bool[])
                n424 = And Array Elements(Boolean array=w1138) -> (logical AND=w1135:bool)
                n425 = case shown="True" w1135 {
                  tunnel: w1153 -> [_ w1169]
                  tunnel: w1152 -> [_ w1168]
                  tunnel: w1151 -> [_ w1167]
                  tunnel: w1150 -> [_ w1166]
                  tunnel: w1149 -> [_ w1165]
                  tunnel: [_ w1164] -> w1148
                  tunnel: w1147 -> [_ w1163]
                  tunnel: w1146 -> [_ w1162]
                  tunnel: [_ w1161] -> w1145
                  tunnel: w1144 -> [_ w1160]
                  tunnel: w1143 -> [_ w1159]
                  tunnel: w1142 -> [_ w1158]
                  tunnel: w1134 -> [_ w1157]
                  tunnel: w1134 -> [_ w1156]
                  frame False {
                    w1154 = "失败" ("布尔文本.文本")
                    w1155 = cluster{u32, u32}[] [{16711680, 0}] ("颜色[4]")
                    n426 = property on="烧录结果" class="Bool (strict)"("Colors [4]"=w1155, "BoolText.Text"=w1154) -> ()  [unwired: 2 in, 2 out]
                    n427 = property on="校验" class="Bool (strict)"("Colors [4]"=w1155, "BoolText.Text"=w1154) -> ()  [unwired: 2 in, 2 out]
                  }
                  frame True {
                    n428 = case shown="True" w1169 {
                      tunnel: w1168 -> [w1182 w1282]
                      tunnel: w1167 -> [w1181 w1281]
                      tunnel: w1166 -> [w1180 w1280]
                      tunnel: w1165 -> [_ w1279]
                      tunnel: w1163 -> [_ w1278]
                      tunnel: [w1179 w1277] -> w1164
                      tunnel: w1163 -> [w1178 _]
                      tunnel: w1162 -> [w1175 _]
                      tunnel: w1160 -> [w1183 _]
                      tunnel: [w1177 w1273] -> w1161
                      tunnel: w1160 -> [w1176 w1273]
                      tunnel: w1159 -> [w1172 w1271]
                      tunnel: w1158 -> [w1171 _]
                      tunnel: w1157 -> [_ w1269]
                      tunnel: w1156 -> [w1170 _]
                      frame False {
                        n429 = Greater?(x=w1175, y=0) -> (0:w1173:bool)
                        n430 = case shown="True" w1173 {
                          tunnel: w1183 -> [_ w1231]
                          tunnel: w1182 -> [w1187 w1234]
                          tunnel: w1181 -> [w1186 w1233]
                          tunnel: w1180 -> [w1190 w1232]
                          tunnel: [w1206 w1230] -> w1179
                          tunnel: w1178 -> [w1206 _]
                          tunnel: [w1205 w1229] -> w1177
                          tunnel: w1176 -> [w1205 _]
                          tunnel: w1172 -> [_ w1222]
                          tunnel: w1171 -> [w1192 _]
                          tunnel: w1170 -> [_ w1220]
                          frame False {
                            w1184 = "成功" ("布尔文本.文本")
                            w1185 = cluster{u32, u32}[] [{6618880, 0}] ("颜色[4]")
                            w1200 = u8 0 ("元素")
                            n431 = flat-sequence {
                              tunnel: w1192 -> [w1217]
                              tunnel: [w1217] -> w1191
                              tunnel: [w1219] -> w1193
                              tunnel: w1191 -> [w1219]
                              frame #0 {
                                n432 = invoke on="开始监控 2" class="Bool" method="Reinit To Default"() -> ()  [unwired: 3 in, 3 out]
                                n433 = local write "TEMP"(FALSE ("TEMP")) -> ()
                              }
                              frame #1 {
                                n434 = Wait (ms)(milliseconds to wait=u32 500 ("等待时间（毫秒）")) -> ()  [unwired: 1 out]
                              }
                            }
                            n435 = Bundle(cluster=w1193, "ID"=u32 0, "TimeStamp"=u8 0 ("RemoteFlag"), "TimeFlag"=u8 1, "SendType"=u8 0 ("DataLen"), "RemoteFlag"=u8 0, "ExternFlag"=u8 0, "DataLen"=u8 1, u8 5 ("元素"), w1200, w1200, w1200) -> (w1204:T2)  [unwired: 7 in]
                            n436 = dll-call lib="PTH2{abs DPCTools2.sourceSNV-AutoTestV1.0.0ASettingsSEQEditDriver平台BCUAutoBurnSettingsControlCAN.dll" fn="VCI_Transmit"("DeviceType"=w1187, "DeviceInd"=w1186, "CANInd"=w1190, "pSend"=w1204, "Len"=u32 1) -> (error out=w1189:errorcluster)  [unwired: 5 in, 5 out]
                            n437 = local read "Mode"() -> (w1188:bool)
                            n438 = case shown="False" w1188 {
                              tunnel: w1187 -> [_ w1215]
                              tunnel: w1186 -> [_ w1214]
                              tunnel: w1190 -> [_ w1213]
                              tunnel: w1189 -> [_ w1211]
                              frame False {
                                n439 = flat-sequence {
                                frame #0 {
                                n440 = Wait (ms)(milliseconds to wait=u32 500 ("等待时间（毫秒）")) -> ()  [unwired: 1 out]
                                }
                                frame #1 {
                                n441 = local write "TEMP"(TRUE ("TEMP")) -> ()
                                n442 = local write "连接状态"(TRUE ("CAN连接状态")) -> ()
                                }
                                }
                              }
                              frame True {
                                n443 = invoke on="开始监控" class="Bool" method="Reinit To Default"() -> ()  [unwired: 3 in, 3 out]
                                n444 = local write "连接状态"(FALSE ("CAN连接状态")) -> ()
                                n445 = call "CAN_Init.vi"("设备类型"=w1215, "设备索引"=w1214, "CAN路数"=w1213, "操作类型"=enum16{"初始化CAN", "关闭CAN"}."关闭CAN", "error in (no error)"=w1211) -> ()  [unwired: 13 in, 2 out]
                              }
                            }
                            n446 = property on="烧录结果" class="Bool (strict)"("Colors [4]"=w1185, "BoolText.Text"=w1184) -> ()  [unwired: 2 in, 2 out]
                            n447 = invoke on="Monitor" class="Bool" method="Reinit To Default"() -> ()  [unwired: 3 in, 3 out]
                            n448 = property on="校验" class="Bool (strict)"("Colors [4]"=w1185, "BoolText.Text"=w1184) -> ()  [unwired: 2 in, 2 out]
                          }
                          frame True {
                            w1224 = 100.0 ("y")
                            n449 = Delete From Array(array=w1231, length=1 ("长度"), index=0 ("索引")) -> (array with subset deleted=w1229:string[])  [unwired: 1 out]
                            n450 = local read "大小"() -> (w1227:i32)
                            n451 = Array Size(array=w1229) -> (size(s)=w1228:i32)
                            n452 = Index Array(array=w1231, index=0 ("索引")) -> (element=w1239:string)
                            n453 = Divide(x=w1228, y=w1227) -> (x/y=w1226:dbl)
                            n454 = String Subset(string=w1239, offset (0)=0 ("偏移量(0)"), length (rest)=2 ("长度（剩余）")) -> (substring=w1246:string)
                            n455 = String Subset(string=w1239, offset (0)=2 ("偏移量(0)"), length (rest)=2 ("长度（剩余）")) -> (substring=w1249:string)
                            n456 = Multiply(x=w1226, y=w1224) -> (x*y=w1225:dbl)
                            n457 = Subtract(x=w1224, y=w1225) -> (x-y=w1223:dbl)
                            n458 = Hexadecimal String To Number(string=w1249) -> (number=w1244:u32)  [unwired: 2 in, 1 out]
                            n459 = case shown="\"S1\", Default" w1246 {
                              tunnel: [4 ("偏移量(0)") 6 ("偏移量(0)")] -> w1238
                              tunnel: w1244 -> [w1261 w1267]
                              tunnel: [w1259 w1265] -> w1243
                              tunnel: [8 ("y") 10 ("y")] -> w1240
                              tunnel: ["S1" "S2"] -> w1235
                              frame "S1", Default {
                                n460 = Subtract(x=w1261, y=3) -> (x-y=w1259:u32)
                              }
                              frame "S2" {
                                n461 = Subtract(x=w1267, y=4) -> (x-y=w1265:u32)
                              }
                            }
                            "地址长度 2" <- w1238
                            n462 = local write "进度"(w1223) -> ()
                            n463 = String Subset(string=w1239, offset (0)=4 ("偏移量(0)"), length (rest)=w1238) -> ()  [unwired: 1 out]
                            n464 = Multiply(x=u32 2, y=w1243) -> (x*y=w1241:u32)
                            "数据长度 2" <- w1241
                            n465 = String Subset(string=w1239, offset (0)=4 ("偏移量(0)"), length (rest)=w1238) -> (substring=w1236:string)
                            n466 = call "CAN R&W.vi"("设备类型"=w1234, "设备索引"=w1233, "CAN路数"=w1232, "DataLen"=u8 8, "写地址/数据"=enum16{"写地址", "写数据"}."写地址", "Data Input"=w1236, "枚举"=w1222, "TYPE"=w1235, "queue out"=w1220) -> ("发送的数据"=w1221:i32[])  [unwired: 17 in, 1 out]
                            n467 = local write "发送的数据"(w1221) -> ()
                            n468 = String Subset(string=w1239, offset (0)=w1240, length (rest)=w1241) -> (substring=w1230:string)
                            "子字符串 2" <- w1230
                          }
                        }
                      }
                      frame True {
                        n469 = Quotient & Remainder(x=w1279, y=12) -> (x-y*floor(x/y)=w1274:i32, floor(x/y)=w1275:i32)
                        n470 = Greater Than 0?(x=w1275) -> (x > 0?=w1284:bool)
                        n471 = case shown="False" w1284 {
                          tunnel: w1278 -> [w1304 w1329]
                          tunnel: w1279 -> [_ w1326]
                          tunnel: ["" w1325] -> w1277
                          tunnel: [w1289 w1324] -> w1272
                          tunnel: w1274 -> [w1302 _]
                          tunnel: [w1290 u8 8 ("DataLen")] -> w1276
                          tunnel: w1273 -> [w1299 _]
                          tunnel: w1271 -> [w1288 _]
                          frame False {
                            n472 = Divide(x=w1302, y=2) -> (x/y=w1287:dbl)
                            n473 = Array Size(array=w1299) -> (size(s)=w1298:i32)
                            n474 = String Subset(string=w1304, length (rest)=w1302) -> (substring=w1292:string)  [unwired: 1 in]
                            n475 = Increment(x=w1287) -> (x+1=w1300:dbl)
                            n476 = Increment(x=w1300) -> (x+1=w1291:dbl)
                            n477 = Equal?(x=0, y=w1298) -> (x = y?=w1286:bool)
                            n478 = Quotient & Remainder(x=w1287, y=2.0) -> (x-y*floor(x/y)=w1295:dbl)  [unwired: 1 out]
                            n479 = local write "发送数据长度"(w1287) -> ()
                            n480 = Equal?(x=w1295, y=1.0) -> (x = y?=w1293:bool)
                            n481 = case shown="True" w1286 {
                              frame False {
                              }
                              frame True {
                                w1305 = "成功" ("布尔文本.文本")
                                w1306 = cluster{u32, u32}[] [{6618880, 0}] ("颜色[4]")
                                n482 = invoke on="Monitor" class="Bool" method="Reinit To Default"() -> ()  [unwired: 3 in, 3 out]
                                n483 = property on="烧录结果" class="Bool (strict)"("Colors [4]"=w1306, "BoolText.Text"=w1305) -> ()  [unwired: 2 in, 2 out]
                                n484 = property on="校验" class="Bool (strict)"("Colors [4]"=w1306, "BoolText.Text"=w1305) -> ()  [unwired: 2 in, 2 out]
                              }
                            }
                            n485 = case shown="False" w1293 {
                              tunnel: w1292 -> [w1307 w1311]
                              tunnel: w1291 -> [w1308 w1313]
                              tunnel: [w1308 w1312] -> w1290
                              tunnel: [w1307 w1310] -> w1289
                              tunnel: w1288 -> [_ w1309]
                              frame False {
                              }
                              frame True {
                                n486 = case shown="\"主板\"" w1309 {
                                tunnel: w1313 -> [w1318 w1320]
                                tunnel: [w1317 w1320] -> w1312
                                tunnel: w1311 -> [w1316 w1319]
                                tunnel: [w1314 w1319] -> w1310
                                frame "主板" {
                                n487 = Concatenate Strings(w1316, "FF") -> (w1314:string)
                                n488 = Increment(x=w1318) -> (x+1=w1317:dbl)
                                }
                                frame "从板", Default {
                                }
                                }
                              }
                            }
                          }
                          frame True {
                            w1323 = 12 ("长度（剩余）")
                            n489 = Subtract(x=w1326, y=12 ("长度（剩余）")) -> (x-y=w1328:i32)
                            n490 = String Subset(string=w1329, offset (0)=w1323, length (rest)=w1328) -> (substring=w1325:string)
                            n491 = String Subset(string=w1329, length (rest)=w1323) -> (substring=w1324:string)  [unwired: 1 in]
                            n492 = local write "发送数据长度"(6.0 ("发送数据长度")) -> ()
                          }
                        }
                        n493 = call "CAN R&W.vi"("设备类型"=w1282, "设备索引"=w1281, "CAN路数"=w1280, "DataLen"=w1276, "写地址/数据"=enum16{"写地址", "写数据"}."写数据", "Data Input"=w1272, "枚举"=w1271, "queue out"=w1269) -> ("发送的数据"=w1270:i32[])  [unwired: 18 in, 1 out]
                        n494 = local write "发送的数据"(w1270) -> ()
                      }
                    }
                  }
                }
              }
              frame Enabled {
              }
            }
          }
          frame 1, Default {
            (unwired) TRUE
            # "040000"
            n495 = local read "请选择板号"() -> (w1334:u16)
            n496 = Increment(x=w1334) -> (x+1=w1333:u16)
            n497 = Subtract(x=w1335, y=w1333) -> (x-y=w1332:u32)
            n498 = case shown="4010000" w1332 {
              tunnel: w1331 -> [_ w1338 w1343]
              tunnel: w1330 -> [_ _ w1342]
              frame 0, Default {
              }
              frame 67108864 {
                n499 = local write "Life"(w1338) -> ()
              }
              frame 67174400 {
                n500 = Join Numbers(hi=w1343, lo=w1342) -> ((hi.lo)=w1341:u16)
                n501 = Divide(x=w1341, y=u16 10) -> (x/y=→"总电压":dbl)
              }
            }
          }
        }
      }
    }
  }
  n502 = stacked-sequence {
    tunnel: "错误输入（无错误）" -> [w1361 w1393 w1504]
    tunnel: [w1356 _ _] -> w1
    frame #0 {
      w1387 = "BURNRESULT" ("section")
      w1391 = u32 21 items=["PCI5121"=1, "PCI9810"=2, "USBCAN1"=3, "USBCAN2"=4, "PCI9820"=5, "CAN232"=6, "PCI5110"=7, "CANLite(mini)"=8, "ISA9620"=9, "ISA5420"=10, "PC104CAN"=11, "CANET"=17, "DNP9810"=13, "USBCAN-E-U"=20, "USBCAN-2E-U"=21] ("类型")
      w1390 = u32 4 items=["PCI5121"=1, "PCI9810"=2, "USBCAN1"=3, "USBCAN2"=4, "PCI9820"=5, "CAN232"=6, "PCI5110"=7, "CANLite(mini)"=8, "ISA9620"=9, "ISA5420"=10, "PC104CAN"=11, "CANET"=17, "DNP9810"=13, "USBCAN-E-U"=20, "USBCAN-2E-U"=21] ("类型")
      # "识别CAN卡，文件路径等"
      n503 = call <vilib>:"Open Config Data.vi"("error in (no error)"=w1361, "configuration file path"=path "D:/BlueWay/configresult.ini") -> ("error out"=w1385:errorcluster, "refnum"=w1388:T4)  [unwired: 7 in, 1 out]
      n504 = call <vilib>:"Open Config Data.vi"("error in (no error)"=w1361, "configuration file path"=path "D:/BlueWay/BMU从板号.ini") -> ("error out"=w1371:errorcluster, "refnum"=w1369:T4)  [unwired: 7 in, 1 out]
      n505 = call <vilib>:"Open Config Data.vi"("error in (no error)"=w1361, "configuration file path"=path "D:/自动测试项目文件/ProjectSetting.ini") -> ("error out"=w1376:errorcluster, "refnum"=w1375:T4)  [unwired: 7 in, 1 out]
      n506 = call-poly <vilib>:"Write Key.vi"("section"=w1387, "error in (no error)"=w1385, "value"="FAIL" ("section"), "key"=w1387, "refnum"=w1388) -> ("error out"=w1383:errorcluster, "refnum out"=w1384:T4)  [unwired: 4 in, 1 out]
      n507 = call <vilib>:"Close Config Data.vi"("error in (no error)"=w1383, "refnum"=w1384) -> ()  [unwired: 8 in, 2 out]
      n508 = Select(t=w1390, s=TRUE, f=w1391) -> (s? t:f=w1392:u32)
      n509 = call-poly <vilib>:"Read Key.vi"("section"="BMUNO", "error in (no error)"=w1371, "key"="BMUNO", "refnum"=w1369) -> ("error out"=w1352:errorcluster, "value"=w1377:string, "refnum out"=w1353:T4)  [unwired: 4 in, 1 out]
      n510 = local write "类型"(w1392) -> ()
      n511 = Decimal String To Number(string=w1377) -> (number=w1360:i32)  [unwired: 2 in, 1 out]
      n512 = local write "请选择板号"(w1360) -> ()
      n513 = call-poly <vilib>:"Read Key.vi"("section"="PROJECT", "error in (no error)"=w1376, "key"="内部CAN波特率", "refnum"=w1375) -> ("error out"=w1357:errorcluster, "value"=w1374:string, "refnum out"=w1379:T4)  [unwired: 4 in, 1 out]
      n514 = call-poly <vilib>:"Read Key.vi"("section"="PROJECT", "error in (no error)"=w1357, "key"="BCU应用程序" ("字符串"), "refnum"=w1379) -> ("error out"=w1356:errorcluster, "value"=w1380:string)  [unwired: 4 in, 2 out]
      n515 = call-poly <vilib>:"Read Key.vi"("section"="BCUTYPE", "error in (no error)"=w1352, "key"="BCUTYPE", "refnum"=w1353) -> ("error out"=w1350:errorcluster, "value"=w1348:string, "refnum out"=w1351:T4)  [unwired: 4 in, 1 out]
      n516 = Equal?(x=w1374, y="500K") -> (x = y?=w1365:bool)
      n517 = Select(t=T1."500Kbps" ("波特率"), s=w1365, f=T1."250Kbps" ("波特率")) -> (s? t:f=w1359:T1)
      n518 = Build Path(base path=path "D:/自动测试项目文件" ("基路径"), name or relative path=w1380) -> (appended path=w1346:path)
      n519 = local write "波特率"(w1359) -> ()
      n520 = Equal?(x=w1348, y="通用") -> (x = y?=w1349:bool)
      n521 = call <vilib>:"Close Config Data.vi"("error in (no error)"=w1350, "refnum"=w1351) -> ()  [unwired: 8 in, 2 out]
      n522 = Select(t=path "D:/BlueWay/通用文件/TYXXXXMSXXXX.s19" ("基路径"), s=w1349, f=w1346) -> (s? t:f=w1344:path)
      n523 = local write "应用程序路径"(w1344) -> ()
    }
    frame #1 {
      n524 = local read "应用程序路径"() -> (w1394:path)
      n525 = Not A Number/Path/Refnum?(number/path/refnum=w1394) -> (NaN/Path/Refnum?=w1398:bool)
      n526 = Strip Path(path=w1394) -> (name=w1401:string)  [unwired: 1 out]
      n527 = String Subset(string=w1401, offset (0)=6 ("偏移量(0)"), length (rest)=2 ("长度（剩余）")) -> (substring=w1397:string)
      n528 = case shown="\"MS\"" w1397 {
        tunnel: [TRUE ("y") FALSE ("y") FALSE ("y")] -> w1400
        frame "假", Default {
          n529 = local read "Info："() -> (w1403:string)
          n530 = Concatenate Strings(w1403, "无法识别板类型！\n" ("字符串")) -> (w1405:string)
          n531 = local write "Info："(w1405) -> ()
        }
        frame "MS" {
          n532 = local read "Info："() -> (w1407:string)
          n533 = local write "目标板类型"(enum16{"BCU/主板", "BMU/从板"}."BCU/主板" ("类型")) -> ()
          n534 = property on="请选择板号" class="Ring (strict)"("Visible"=FALSE ("可见")) -> ()  [unwired: 2 in, 2 out]
          n535 = Concatenate Strings(w1407, "通过文件识别为主板！\n" ("字符串")) -> (w1408:string)
          n536 = local write "Info："(w1408) -> ()
        }
        frame "SS" {
          n537 = local read "Info："() -> (w1413:string)
          n538 = local write "目标板类型"(enum16{"BCU/主板", "BMU/从板"}."BMU/从板" ("类型")) -> ()
          n539 = property on="请选择板号" class="Ring (strict)"("Visible"=TRUE ("可见")) -> ()  [unwired: 2 in, 2 out]
          n540 = Concatenate Strings(w1413, "通过文件识别为从板！\n" ("字符串")) -> (w1414:string)
          n541 = local write "Info："(w1414) -> ()
        }
      }
      n542 = Or(x=w1398, y=w1400) -> (x .or. y?=w1399:bool)
      n543 = case shown="False" w1399 {
        tunnel: w1394 -> [w1454 _]
        tunnel: w1393 -> [w1418 _]
        frame False {
          n544 = Path To String(path=w1454) -> (string=w1429:string)
          n545 = local read "Info："() -> (w1425:string)
          n546 = String Subset(string=w1429, offset (0)=6 ("偏移量(0)"), length (rest)=2 ("长度（剩余）")) -> (substring=w1426:string)
          n547 = call-poly <vilib>:"Read From Spreadsheet File.vi"("file path (dialog if empty)"=w1454) -> ("all rows"=w1456:string[][])  [unwired: 6 in, 4 out]
          n548 = call <vilib>:"Space Constant.vi"() -> ("String"=w1452:string)
          n549 = Search and Replace String(replace all?=TRUE ("替换全部？(F)"), input string=w1429, search string=w1452, replace string="" ("替换字符串(\"\")")) -> (result string=w1439:string)  [unwired: 4 in, 3 out]
          n550 = case shown="\"真\"" w1426 {
            frame "假", Default {
            }
            frame "真" {
            }
          }
          n551 = Concatenate Strings(w1425, "文件加载成功！\n" ("字符串")) -> (w1423:string)
          n552 = Index Array(array=w1456, index (col)=0 ("禁用的索引 (列)")) -> (element=w1443:string[])  [unwired: 1 in]
          n553 = Search/Split String(string=w1439, search string/char (-)="(MD5=" ("搜索字符串/字符(-)")) -> (match + rest of string=w1436:string, offset of match=w1446:i32)  [unwired: 1 in, 1 out]
          n554 = local write "Info："(w1423) -> ()
          n555 = Delete From Array(array=w1443, length=1 ("长度"), index=0 ("索引")) -> (array with subset deleted=w1435:string[])  [unwired: 1 out]
          n556 = call <vilib>:"MD5Checksum File.vi"("error in (no error)"=w1418, "Path"=w1454) -> ("MD5 message-digest"=w1420:string)  [unwired: 8 in, 1 out]
          n557 = Array Size(array=w1435) -> (size(s)=w1433:i32)
          n558 = Decrement(x=w1433) -> (x-1=w1432:i32)
          n559 = Delete From Array(array=w1435, length=1 ("长度"), index=w1432) -> (array with subset deleted=w1431:string[])  [unwired: 1 out]
          n560 = Array Size(array=w1431) -> (size(s)=w1419:i32)
          n561 = local write "校验码实际值"(w1420) -> ()
          n562 = Add(x=w1446, y=5) -> (x+y=w1447:i32)
          n563 = Search/Split String(string=w1439, search string/char (-)=")" ("搜索字符串/字符(-)")) -> ()  [unwired: 1 in, 3 out]
          n564 = String Subset(string=w1436, offset (0)=45 ("偏移量(0)"), length (rest)=8 ("长度（剩余）")) -> ()  [unwired: 1 out]
          n565 = local write "总行数"(w1419) -> ()
          n566 = String Subset(string=w1439, offset (0)=w1447, length (rest)=32 ("长度（剩余）")) -> (substring=w1437:string)
          n567 = Equal?(x=w1437, y=w1420) -> (x = y?=w1444:bool)
          n568 = case shown="True" w1444 {
            frame False {
              n569 = Build Array(cluster{u32, u32} {16711680, 0}) -> (w1486:cluster{u32, u32}[])
              n570 = property on="MD5校验" class="Bool (strict)"("Colors [4]"=w1486, "BoolText.Text"="失败" ("布尔文本.文本")) -> ()  [unwired: 2 in, 2 out]
            }
            frame True {
              n571 = Build Array(cluster{u32, u32} {6618880, 0}) -> (w1489:cluster{u32, u32}[])
              n572 = property on="MD5校验" class="Bool (strict)"("Colors [4]"=w1489, "BoolText.Text"="成功" ("布尔文本.文本")) -> ()  [unwired: 2 in, 2 out]
            }
          }
          n573 = local write "校验码期望值"(w1437) -> ()
          n574 = for {
            tunnel: w1431 -> [w1467] mode=indexing
            shift-right: [w1465] -> w1421
            shift-left: u16 0 ("偏移量(0)") -> [w1466]
            tunnel: [w1459] -> w1422 mode=indexing
            n575 = String Subset(string=w1467, offset (0)=1 ("偏移量(0)"), length (rest)=1 ("长度（子字符串长度）")) -> (substring=w1470:string)
            n576 = case shown="\"1\", Default" w1470 {
              tunnel: ["01" ("子字符串(\"\")") "02" ("子字符串(\"\")")] -> w1471
              frame "1", Default {
              }
              frame "2" {
              }
            }
            n577 = String Subset(string=w1467, offset (0)=2 ("偏移量(0)")) -> (substring=w1473:string)  [unwired: 1 in]
            n578 = Concatenate Strings("FFFFFFFFFFFF" ("子字符串(\"\")"), w1471, w1473) -> (w1459:string)
            n579 = String Subset(string=w1459, offset (0)=12 ("偏移量(0)")) -> (substring=w1457:string)  [unwired: 1 in]
            n580 = String Length(string=w1457) -> (length=w1464:i32)
            n581 = Divide(x=w1464, y=2) -> (x/y=w1462:dbl)
            n582 = for {
              N: w1462 -> [_]
              tunnel: w1457 -> [w1482]
              shift-right: [w1477] -> w1460
              shift-left: u16 0 ("偏移量(0)") -> [w1475]
              i -> [w1481]
              w1479 = 2 ("x")
              n583 = Multiply(x=w1479, y=w1481) -> (x*y=w1480:i32)
              n584 = String Subset(string=w1482, offset (0)=w1480, length (rest)=w1479) -> (substring=w1478:string)
              n585 = call "ASCII_To_Hex.vi"("ASCII String"=w1478) -> ("hex1"=w1476:u8)  [unwired: 6 in, 4 out]
              n586 = Add(x=w1475, y=w1476) -> (x+y=w1477:u16)
            }
            n587 = Add(x=w1466, y=w1460) -> (x+y=w1465:u16)
          }
          n588 = local write "CRC16"(w1421) -> ()
          n589 = local write "子数组"(w1422) -> ()
        }
        frame True {
          n590 = flat-sequence {
            frame #0 {
              n591 = local read "Info："() -> (w1492:string)
              n592 = Concatenate Strings(w1492, "文件加载错误！\n" ("字符串")) -> (w1491:string)
              n593 = local write "Info："(w1491) -> ()
            }
            frame #1 {
              n594 = Wait (ms)(milliseconds to wait=u32 2000 ("等待时间（毫秒）")) -> ()  [unwired: 1 out]
            }
            frame #2 {
              n595 = local read "设备索引"() -> (w1496:u32)
              n596 = local read "CAN路数"() -> (w1498:u32)
              n597 = local read "波特率"() -> (w1497:T1)
              n598 = local read "滤波方式"() -> (w1499:u8)
              n599 = local read "工作方式"() -> (w1500:u8)
              n600 = local read "类型"() -> (w1495:u32)
              n601 = call "CAN_Init.vi"("设备类型"=w1495, "设备索引"=w1496, "波特率"=w1497, "CAN路数"=w1498, "操作类型"=enum16{"初始化CAN", "关闭CAN"}."关闭CAN", "滤波方式"=w1499, "工作方式"=w1500) -> ()  [unwired: 11 in, 2 out]
            }
            frame #3 {
              n602 = Quit LabVIEW(quit? (T)=TRUE ("退出？(T)")) -> ()
            }
          }
        }
      }
    }
    frame #2 {
      w1508 = "" ("布尔文本.文本")
      w1509 = cluster{u32, u32}[] [{0, 0}] ("颜色[4]")
      w1510 = FALSE
      n603 = local write "update flag"(TRUE ("update flag")) -> ()
      n604 = property on="烧录结果" class="Bool (strict)"("Colors [4]"=w1509, "BoolText.Text"=w1508) -> ()  [unwired: 2 in, 2 out]
      n605 = local read "设备索引"() -> (w1517:u32)
      n606 = local read "CAN路数"() -> (w1515:u32)
      n607 = local read "波特率"() -> (w1516:T1)
      n608 = local read "滤波方式"() -> (w1514:u8)
      n609 = local read "工作方式"() -> (w1513:u8)
      n610 = local read "类型"() -> (w1518:u32)
      n611 = property on="校验" class="Bool (strict)"("Colors [4]"=w1509, "BoolText.Text"=w1508) -> ()  [unwired: 2 in, 2 out]
      n612 = call "CAN_Init.vi"("设备类型"=w1518, "设备索引"=w1517, "波特率"=w1516, "CAN路数"=w1515, "操作类型"=enum16{"初始化CAN", "关闭CAN"}."初始化CAN", "error in (no error)"=w1504, "滤波方式"=w1514, "工作方式"=w1513) -> ("CAN 操作结果"=w1506:bool, "error out"=w1503:errorcluster)  [unwired: 10 in]
      n613 = local write "擦除完成"(w1510) -> ()
      n614 = local write "进度"(u8 0 ("进度")) -> ()
      n615 = local write "进入烧录模式"(w1510) -> ()
      n616 = local write "烧录结果"(w1510) -> ()
      n617 = local write "Monitor_flag"(FALSE ("Monitor_flag")) -> ()
      n618 = local write "CAN状态"(w1506) -> ()
      n619 = local write "连接状态"(w1506) -> ()
      n620 = case shown="True" w1506 {
        tunnel: w1504 -> [w1519 _]
        tunnel: w1503 -> [_ _]
        frame True {
          n621 = local read "Info："() -> (w1520:string)
          n622 = stacked-sequence {
            tunnel: w1519 -> [w1528 _ _]
            tunnel: [w1527 _ _] -> _
            frame #0 {
              n623 = disable-structure shown="启用" {
                disable-tunnel: w1528 -> [w1531 _]
                disable-tunnel: [w1530 _] -> w1527
                frame Enabled {
                  n624 = local read "CAN路数"() -> (w1532:u32)
                  n625 = local read "设备索引"() -> (w1533:u32)
                  n626 = local read "类型"() -> (w1534:u32)
                  n627 = dll-call lib="PTH2{abs DPCTools2.sourceSNV-AutoTestV1.0.0ASettingsSEQEditDriver平台BCUAutoBurnSettingsControlCAN.dll" fn="VCI_ClearBuffer" label="VCI_Clearbuffer"(error in=w1531, "DeviceType"=w1534, "DeviceInd"=w1533, "CANInd"=w1532) -> (error out=w1530:errorcluster)  [unwired: 3 in, 4 out]
                }
                frame Disabled {
                }
              }
              n628 = local write "boot模式应答...成功"(FALSE) -> ()
              n629 = local write "开始下载数据"(FALSE ("开始下载数据")) -> ()
              n630 = local write "进入烧录"(TRUE ("布尔")) -> ()
              n631 = local write "开始下载数据"(u32 0 ("开始下载数据")) -> ()
            }
            frame #1 {
              w1540 = TRUE ("T1")
              w1539 = TRUE ("T1")
              n632 = local read "Info："() -> (w1535:string)
              n633 = Concatenate Strings(w1535, "boot模式请求..." ("字符串"), "\n") -> (w1538:string)
              n634 = local write "Info："(w1538) -> ()
              n635 = local write "T2"(w1539) -> ()
              n636 = local write "T3"(w1540) -> ()
              n637 = local write "T1"(w1539) -> ()
              n638 = local write "T4"(w1540) -> ()
              n639 = local write "T5"(w1540) -> ()
              n640 = local write "T6"(w1540) -> ()
              n641 = local write "T7"(w1540) -> ()
              n642 = local write "T8"(u8 0 ("T8")) -> ()
              n643 = local write "T9"(w1540) -> ()
            }
            frame #2 {
              n644 = local read "目标板类型"() -> (w1544:enum16{"BCU/主板", "BMU/从板"})
              n645 = case shown="\"BCU/主板\", Default" w1544 {
                tunnel: [u16 0 ("请选择板号") w1557] -> w1545
                frame "BCU/主板", Default {
                }
                frame "BMU/从板" {
                  n646 = local read "请选择板号"() -> (w1557:u16)
                }
              }
              n647 = Tick Count (ms)() -> (millisecond timer value=w1543:u32)
              n648 = local write "start"(w1543) -> ()
              n649 = local write "boot模式应答计数"(0 ("boot模式应答计数")) -> ()
              n650 = Multiply(x=w1545, y=u16 256) -> (x*y=w1548:u16)
              n651 = Add(x=u32 65681 ("ID"), y=w1548) -> (x+y=w1546:u32)
              n652 = local read "VCI_CAN_OBJ_T"() -> (w1550:T2)
              n653 = case shown="1, Default" w1545 {
                tunnel: [w1562 w1574] -> w1554
                tunnel: w1550 -> [w1561 w1573]
                tunnel: w1546 -> [w1559 w1571]
                frame 0 {
                  w1558 = u8 170
                  w1565 = u8 0 ("元素")
                  n654 = Bundle(cluster=w1561, "ID"=w1559, "TimeStamp"=u8 0 ("RemoteFlag"), "TimeFlag"=u8 1, "SendType"=u8 0 ("DataLen"), "RemoteFlag"=u8 0, "ExternFlag"=u8 1, "DataLen"=u8 8, u8 1 ("元素"), w1558, w1558, w1558, w1558, w1565, w1565, w1565) -> (w1562:T2)  [unwired: 3 in]
                }
                frame 1, Default {
                  w1570 = u8 187
                  w1577 = u8 0 ("元素")
                  n655 = Bundle(cluster=w1573, "ID"=w1571, "TimeStamp"=u8 0 ("RemoteFlag"), "TimeFlag"=u8 1, "SendType"=u8 0 ("DataLen"), "RemoteFlag"=u8 0, "ExternFlag"=u8 1, "DataLen"=u8 8, u8 1 ("元素"), w1570, w1570, w1570, w1570, w1577, w1577, w1577) -> (w1574:T2)  [unwired: 3 in]
                }
              }
              n656 = local read "设备索引"() -> (w1552:u32)
              n657 = local read "CAN路数"() -> (w1551:u32)
              n658 = local read "类型"() -> (w1553:u32)
              n659 = dll-call lib="PTH2{abs DPCTools2.sourceSNV-AutoTestV1.0.0ASettingsSEQEditDriver平台BCUAutoBurnSettingsControlCAN.dll" fn="VCI_Transmit"("DeviceType"=w1553, "DeviceInd"=w1552, "CANInd"=w1551, "pSend"=w1554, "Len"=u32 1) -> ()  [unwired: 5 in, 6 out]
            }
          }
          n660 = Concatenate Strings(w1520, "启动CAN成功.." ("字符串"), "\n") -> (w1523:string)
          n661 = local write "Info："(w1523) -> ()
        }
        frame False {
          n662 = stacked-sequence {
            frame #0 {
              n663 = local read "Info："() -> (w1582:string)
              n664 = Concatenate Strings(w1582, "启动CAN失败.." ("字符串"), "\n") -> (w1585:string)
              n665 = local write "Info："(w1585) -> ()
            }
            frame #1 {
              n666 = local read "设备索引"() -> (w1588:u32)
              n667 = local read "CAN路数"() -> (w1590:u32)
              n668 = local read "波特率"() -> (w1589:T1)
              n669 = local read "滤波方式"() -> (w1591:u8)
              n670 = local read "工作方式"() -> (w1592:u8)
              n671 = local read "类型"() -> (w1587:u32)
              n672 = Wait (ms)(milliseconds to wait=u32 2000 ("等待时间（毫秒）")) -> ()  [unwired: 1 out]
              n673 = call "CAN_Init.vi"("设备类型"=w1587, "设备索引"=w1588, "波特率"=w1589, "CAN路数"=w1590, "操作类型"=enum16{"初始化CAN", "关闭CAN"}."关闭CAN", "滤波方式"=w1591, "工作方式"=w1592) -> ()  [unwired: 11 in, 2 out]
            }
            frame #2 {
              n674 = Quit LabVIEW(quit? (T)=TRUE ("退出？(T)")) -> ()
            }
          }
        }
      }
    }
  }
  n675 = while {
    tunnel: w20 -> [w1600]
    tunnel: [w1599] -> w3
    tunnel: w1 -> [w1598]
    tunnel: [w1597] -> w2
    tunnel: w19 -> [w1595]
    stop <- "停止 2" stop-if-true
    n676 = local read "连接状态"() -> (w1596:bool)
    n677 = case shown="True" w1596 {
      tunnel: w1600 -> [w1608 w1627]
      tunnel: [w1608 w1626] -> w1599
      tunnel: w1598 -> [w1603 w1625]
      tunnel: [w1603 w1624] -> w1597
      tunnel: [w1602 _] -> _
      tunnel: w1595 -> [_ w1612]
      frame False {
        n678 = local read "设备索引"() -> (w1605:u32)
        n679 = local read "CAN路数"() -> (w1604:u32)
        n680 = local read "类型"() -> (w1606:u32)
        n681 = dll-call lib="PTH2{abs DPCTools2.sourceSNV-AutoTestV1.0.0ASettingsSEQEditDriver平台BCUAutoBurnSettingsControlCAN.dll" fn="VCI_ClearBuffer" label="VCI_Clearbuffer"(error in=w1603, "DeviceType"=w1606, "DeviceInd"=w1605, "CANInd"=w1604) -> (error out=w1602:errorcluster)  [unwired: 3 in, 4 out]
        n682 = Wait (ms)(milliseconds to wait=u32 50 ("等待时间（毫秒）")) -> ()  [unwired: 1 out]
      }
      frame True {
        (unwired) TRUE
        n683 = local read "CAN路数"() -> (w1614:u32)
        n684 = local read "设备索引"() -> (w1615:u32)
        n685 = local read "类型"() -> (w1616:u32)
        n686 = dll-call lib="PTH2{abs DPCTools2.sourceSNV-AutoTestV1.0.0ASettingsSEQEditDriver平台BCUAutoBurnSettingsControlCAN.dll" fn="VCI_Receive"(error in=w1625, "DeviceType"=w1616, "DeviceInd"=w1615, "CANInd"=w1614, "pReceive"=w1612, "Len"=u32 1, "WaitTime"=10) -> (error out=w1619:errorcluster, "返回类型"=w1620:u32, "pReceive"=w1618:T2)  [unwired: 7 in, 1 out]
        "接收" <- w1618
        n687 = Equal?(x=w1620, y=1) -> (x = y?=w1609:bool)
        n688 = Unbundle(w1618) -> ("ID"=w1610:u32, w1613:u8)  [unwired: 16 out]
        "ID" <- w1610
        "返回类型" <- w1610
        n689 = Equal?(x=u32 4, y=w1610) -> (x = y?=w1611:bool)
        n690 = And(x=w1611, y=w1609) -> ()  [unwired: 1 out]
        n691 = case shown="True" w1609 {
          tunnel: w1627 -> [w1629 w1640]
          tunnel: [w1629 w1639] -> w1626
          tunnel: w1618 -> [_ w1638]
          tunnel: w1619 -> [w1628 w1637]
          tunnel: [w1628 w1636] -> w1624
          tunnel: w1613 -> [_ w1633]
          tunnel: w1616 -> [_ w1632]
          tunnel: w1615 -> [_ w1631]
          tunnel: w1614 -> [_ w1630]
          frame False {
          }
          frame True {
            n692 = disable-structure shown="禁用" {
              disable-tunnel: w1633 -> [w1646 _]
              disable-tunnel: w1632 -> [w1644 _]
              disable-tunnel: w1631 -> [w1643 _]
              disable-tunnel: w1630 -> [w1642 _]
              frame Disabled {
                n693 = Equal?(x=w1646, y=255) -> (x = y?=w1641:bool)
                n694 = case shown="True" w1641 {
                  tunnel: w1644 -> [_ w1651]
                  tunnel: w1643 -> [_ w1650]
                  tunnel: w1642 -> [_ w1649]
                  frame False {
                  }
                  frame True {
                    n695 = dll-call lib="PTH2{abs DPCTools2.sourceSNV-AutoTestV1.0.0ASettingsSEQEditDriver平台BCUAutoBurnSettingsControlCAN.dll" fn="VCI_Transmit"("DeviceType"=w1651, "DeviceInd"=w1650, "CANInd"=w1649, "pSend"=T2 {"ID"=0, "TimeStamp"=0, "TimeFlag"=1, "SendType"=0, "RemoteFlag"=0, "ExternFlag"=0, "DataLen"=1, 1, 0, 0, 0, 0, 0, 0, 0, 0, 0, 0} ("输出簇 2"), "Len"=u32 1) -> ()  [unwired: 5 in, 6 out]
                  }
                }
              }
              frame Enabled {
              }
            }
            n696 = local read "CAN数据"() -> (w1635:bool)
            n697 = Enqueue Element(queue=w1640, element=w1638, error in (no error)=w1637) -> (queue out=w1639:refnum<queue>, error out=w1636:errorcluster)  [unwired: 1 in, 1 out]
            n698 = Not(x=w1635) -> (.not. x?=w1634:bool)
            n699 = local write "CAN数据"(w1634) -> ()
          }
        }
      }
    }
  }
  n700 = while {
    tunnel: w1 -> [w1652]
    tunnel: w20 -> [w1654]
    tunnel: w1 -> [_]
    stop <- "停止" stop-if-true
    n701 = event shown="[0] Timeout" {
      selector: _ -> [_ _ _ _ _ _ _ _ _ _ _]
      dyn-events: _ -> [_ _ _ _ _ _ _ _ _ _ _]
      timeout: 200 -> [_ _ _ _ _ _ _ _ _ _ _]
      tunnel: w1652 -> [_ w1769 _ _ w1829 _ _ _ _ _ _]
      tunnel: w1654 -> [_ _ _ _ _ _ _ _ w1942 _ _]
      event Timeout {
        n702 = event-data() -> ()  [unwired: 1 in, 2 out]
        n703 = local read "开始下载数据"() -> (w1663:bool)
        n704 = local read "update flag"() -> (w1664:bool)
        n705 = case shown="True" w1664 {
          frame False {
          }
          frame True {
            n706 = local read "start"() -> (w1697:u32)
            n707 = Tick Count (ms)() -> (millisecond timer value=w1698:u32)
            n708 = Subtract(x=w1698, y=w1697) -> (x-y=w1696:u32)
            n709 = local read "目标板类型"() -> (w1694:enum16{"BCU/主板", "BMU/从板"})
            n710 = Divide(x=w1696, y=u32 1000) -> (x/y=w1693:dbl)
            "耗时：" <- w1693
            n711 = To Unsigned Long Integer(number=w1693) -> (unsigned 32bit integer=w1692:u32)
            n712 = case shown="\"BCU/主板\", Default" w1694 {
              tunnel: w1692 -> [w1701 w1717]
              frame "BCU/主板", Default {
                n713 = Equal?(x=w1701, y=80.0) -> (x = y?=w1699:bool)
                n714 = case shown="True" w1699 {
                  frame False {
                  }
                  frame True {
                    n715 = local read "Info："() -> (w1703:string)
                    n716 = local write "update flag"(FALSE ("update flag")) -> ()
                    n717 = Concatenate Strings(w1703, "超时请重试" ("字符串")) -> (w1704:string)
                    n718 = local write "Info："(w1704) -> ()
                    n719 = flat-sequence {
                      frame #0 {
                        n720 = local read "设备索引"() -> (w1712:u32)
                        n721 = local read "CAN路数"() -> (w1710:u32)
                        n722 = local read "波特率"() -> (w1711:T1)
                        n723 = local read "滤波方式"() -> (w1709:u8)
                        n724 = local read "工作方式"() -> (w1708:u8)
                        n725 = local read "类型"() -> (w1713:u32)
                        n726 = call "CAN_Init.vi"("设备类型"=w1713, "设备索引"=w1712, "波特率"=w1711, "CAN路数"=w1710, "操作类型"=enum16{"初始化CAN", "关闭CAN"}."关闭CAN", "滤波方式"=w1709, "工作方式"=w1708) -> ()  [unwired: 11 in, 2 out]
                        n727 = Wait (ms)(milliseconds to wait=u32 2000 ("等待时间（毫秒）")) -> ()  [unwired: 1 out]
                      }
                      frame #1 {
                        n728 = Quit LabVIEW(quit? (T)=TRUE ("退出？(T)")) -> ()
                      }
                    }
                  }
                }
              }
              frame "BMU/从板" {
                n729 = Equal?(x=w1717, y=50.0) -> (x = y?=w1715:bool)
                n730 = case shown="True" w1715 {
                  frame False {
                  }
                  frame True {
                    n731 = local read "Info："() -> (w1719:string)
                    n732 = local write "update flag"(FALSE ("update flag")) -> ()
                    n733 = Concatenate Strings(w1719, "超时请重试\n" ("字符串")) -> (w1720:string)
                    n734 = local write "Info："(w1720) -> ()
                    n735 = flat-sequence {
                      frame #0 {
                        n736 = local read "设备索引"() -> (w1728:u32)
                        n737 = local read "CAN路数"() -> (w1726:u32)
                        n738 = local read "波特率"() -> (w1727:T1)
                        n739 = local read "滤波方式"() -> (w1725:u8)
                        n740 = local read "工作方式"() -> (w1724:u8)
                        n741 = local read "类型"() -> (w1729:u32)
                        n742 = call "CAN_Init.vi"("设备类型"=w1729, "设备索引"=w1728, "波特率"=w1727, "CAN路数"=w1726, "操作类型"=enum16{"初始化CAN", "关闭CAN"}."关闭CAN", "滤波方式"=w1725, "工作方式"=w1724) -> ()  [unwired: 11 in, 2 out]
                        n743 = Wait (ms)(milliseconds to wait=u32 2000 ("等待时间（毫秒）")) -> ()  [unwired: 1 out]
                      }
                      frame #1 {
                        n744 = Quit LabVIEW(quit? (T)=TRUE ("退出？(T)")) -> ()
                      }
                    }
                  }
                }
              }
            }
          }
        }
        n745 = case shown="True" w1663 {
          frame False {
          }
          frame True {
            n746 = local read "开始下载数据"() -> (w1677:u32)
            n747 = Tick Count (ms)() -> (millisecond timer value=w1678:u32)
            n748 = Subtract(x=w1678, y=w1677) -> (x-y=w1676:u32)
            n749 = Divide(x=w1676, y=u32 1000) -> (x/y=w1672:dbl)
            n750 = To Unsigned Long Integer(number=w1672) -> (unsigned 32bit integer=w1671:u32)
            n751 = Equal?(x=w1671, y=3.0) -> (x = y?=w1673:bool)
            n752 = case shown="True" w1673 {
              frame False {
              }
              frame True {
                n753 = flat-sequence {
                  frame #0 {
                    n754 = local read "Info："() -> (w1681:string)
                    n755 = local write "update flag"(FALSE ("update flag")) -> ()
                    n756 = Concatenate Strings(w1681, "数据传输中断！\n" ("字符串")) -> (w1680:string)
                    n757 = local write "Info："(w1680) -> ()
                  }
                  frame #1 {
                  }
                  frame #2 {
                    n758 = local read "设备索引"() -> (w1689:u32)
                    n759 = local read "CAN路数"() -> (w1687:u32)
                    n760 = local read "波特率"() -> (w1688:T1)
                    n761 = local read "滤波方式"() -> (w1686:u8)
                    n762 = local read "工作方式"() -> (w1685:u8)
                    n763 = local read "类型"() -> (w1690:u32)
                    n764 = call "CAN_Init.vi"("设备类型"=w1690, "设备索引"=w1689, "波特率"=w1688, "CAN路数"=w1687, "操作类型"=enum16{"初始化CAN", "关闭CAN"}."关闭CAN", "滤波方式"=w1686, "工作方式"=w1685) -> ()  [unwired: 11 in, 2 out]
                    n765 = Wait (ms)(milliseconds to wait=u32 2000 ("等待时间（毫秒）")) -> ()  [unwired: 1 out]
                  }
                  frame #3 {
                    n766 = Quit LabVIEW(quit? (T)=TRUE ("退出？(T)")) -> ()
                  }
                }
              }
            }
          }
        }
        n767 = local read "boot模式应答...成功"() -> (w1667:bool)
        n768 = local read "进入烧录"() -> (w1665:bool)
        n769 = local read "boot模式应答计数"() -> (w1670:i32)
        n770 = Increment(x=w1670) -> (x+1=w1658:i32)
        n771 = Equal?(x=w1658, y=7) -> (x = y?=w1657:bool)
        n772 = Equal?(x=25.0, y=w1658) -> (x = y?=w1656:bool)
        n773 = Equal?(x=w1658, y=25) -> ()  [unwired: 1 out]
        n774 = Equal?(x=35 ("y"), y=w1658) -> ()  [unwired: 1 out]
        n775 = Not(x=w1667) -> (.not. x?=w1666:bool)
        n776 = Compound Arithmetic op=OR(w1657, w1656) -> (w1661:bool)
        n777 = local write "boot模式应答计数"(w1658) -> ()
        n778 = Compound Arithmetic op=AND(w1661, w1666, w1665) -> (w1668:bool)
        "?" <- w1668
        n779 = case shown="True" w1668 {
          frame False {
          }
          frame True {
            n780 = local read "目标板类型"() -> (w1732:enum16{"BCU/主板", "BMU/从板"})
            n781 = case shown="\"BMU/从板\"" w1732 {
              tunnel: [u16 0 ("请选择板号") w1744] -> w1731
              frame "BCU/主板", Default {
              }
              frame "BMU/从板" {
                n782 = local read "请选择板号"() -> (w1744:u16)
              }
            }
            n783 = Multiply(x=w1731, y=u16 256) -> (x*y=w1735:u16)
            n784 = Add(x=u32 65681 ("ID"), y=w1735) -> (x+y=w1733:u32)
            n785 = local read "VCI_CAN_OBJ_T"() -> (w1737:T2)
            n786 = case shown="1, Default" w1731 {
              tunnel: [w1749 w1761] -> w1741
              tunnel: w1737 -> [w1748 w1760]
              tunnel: w1733 -> [w1746 w1758]
              frame 0 {
                w1745 = u8 170
                w1752 = u8 0 ("元素")
                n787 = Bundle(cluster=w1748, "ID"=w1746, "TimeStamp"=u8 0 ("RemoteFlag"), "TimeFlag"=u8 1, "SendType"=u8 0 ("DataLen"), "RemoteFlag"=u8 0, "ExternFlag"=u8 1, "DataLen"=u8 8, u8 1 ("元素"), w1745, w1745, w1745, w1745, w1752, w1752, w1752) -> (w1749:T2)  [unwired: 3 in]
              }
              frame 1, Default {
                w1757 = u8 187
                w1764 = u8 0 ("元素")
                n788 = Bundle(cluster=w1760, "ID"=w1758, "TimeStamp"=u8 0 ("RemoteFlag"), "TimeFlag"=u8 1, "SendType"=u8 0 ("DataLen"), "RemoteFlag"=u8 0, "ExternFlag"=u8 1, "DataLen"=u8 8, u8 1 ("元素"), w1757, w1757, w1757, w1757, w1764, w1764, w1764) -> (w1761:T2)  [unwired: 3 in]
              }
            }
            n789 = local read "设备索引"() -> (w1739:u32)
            n790 = local read "CAN路数"() -> (w1738:u32)
            n791 = local read "类型"() -> (w1740:u32)
            n792 = dll-call lib="PTH2{abs DPCTools2.sourceSNV-AutoTestV1.0.0ASettingsSEQEditDriver平台BCUAutoBurnSettingsControlCAN.dll" fn="VCI_Transmit"("DeviceType"=w1740, "DeviceInd"=w1739, "CANInd"=w1738, "pSend"=w1741, "Len"=u32 1) -> ()  [unwired: 5 in, 6 out]
          }
        }
      }
      event "开始监控": Value Change {
        n793 = event-data() -> ("NewVal"=w1773:bool)  [unwired: 1 in, 5 out]
        n794 = local write "TEMP"(w1773) -> ()
        n795 = local read "通信端口:"() -> (w1770:u32)
        n796 = local read "CANET地址格式如：192.168.0.178"() -> (w1772:string)
        n797 = local read "设备索引"() -> (w1775:u32)
        n798 = local read "CAN路数"() -> (w1777:u32)
        n799 = local read "波特率"() -> (w1776:T1)
        n800 = local read "滤波方式"() -> (w1778:u8)
        n801 = local read "工作方式"() -> (w1779:u8)
        n802 = local read "类型"() -> (w1774:u32)
        n803 = local read "PC端-协议类型 2"() -> (w1771:enum16{"TCP服务器Server", "TCP客户端Client"})
        n804 = case shown="True" w1773 {
          tunnel: w1774 -> [w1798 w1822]
          tunnel: w1775 -> [w1797 w1821]
          tunnel: w1776 -> [w1796 w1820]
          tunnel: w1777 -> [w1795 w1819]
          tunnel: w1778 -> [w1793 w1817]
          tunnel: w1779 -> [w1792 w1816]
          tunnel: w1772 -> [w1786 w1814]
          tunnel: w1771 -> [w1785 w1813]
          tunnel: w1770 -> [w1784 w1812]
          tunnel: w1769 -> [w1783 _]
          frame True {
            w1780 = T3."Enabled" ("禁用")
            w1788 = "" ("布尔文本.文本")
            w1789 = cluster{u32, u32}[] [{0, 0}] ("颜色[4]")
            w1790 = FALSE
            n805 = call "CAN_Init.vi"("设备类型"=w1798, "设备索引"=w1797, "波特率"=w1796, "CAN路数"=w1795, "操作类型"=enum16{"初始化CAN", "关闭CAN"}."初始化CAN", "error in (no error)"=w1783, "滤波方式"=w1793, "IP"=w1786, "port"=w1784, "工作方式"=w1792, "PC端-协议类型"=w1785) -> ("CAN 操作结果"=w1781:bool, "error out"=w1782:errorcluster)  [unwired: 7 in]
            n806 = local write "Monitor_flag"(FALSE ("Monitor_flag")) -> ()
            n807 = invoke on="Monitor" class="Bool" method="Reinit To Default"(error in=w1782) -> ()  [unwired: 2 in, 3 out]
            n808 = local write "进度"(u8 0 ("进度")) -> ()
            n809 = local write "CAN状态"(w1781) -> ()
            n810 = local write "连接状态"(w1781) -> ()
            n811 = local write "擦除完成"(w1790) -> ()
            n812 = local write "进入烧录模式"(w1790) -> ()
            n813 = property on="烧录结果" class="Bool (strict)"("Colors [4]"=w1789, "BoolText.Text"=w1788) -> ()  [unwired: 2 in, 2 out]
            n814 = property on="校验" class="Bool (strict)"("Colors [4]"=w1789, "BoolText.Text"=w1788) -> ()  [unwired: 2 in, 2 out]
            n815 = local write "烧录结果"(w1790) -> ()
            n816 = case shown="True" w1781 {
              frame True {
                n817 = local read "Info："() -> (w1799:string)
                n818 = Concatenate Strings(w1799, "启动CAN成功.." ("字符串"), "\n") -> (w1802:string)
                n819 = local write "Info："(w1802) -> ()
              }
              frame False {
                n820 = local read "Info："() -> (w1803:string)
                n821 = Concatenate Strings(w1803, "启动CAN失败.." ("字符串"), "\n") -> (w1806:string)
                n822 = local write "Info："(w1806) -> ()
              }
            }
            n823 = property on="手动进入编程模式" class="Bool (strict)"("DisabledEnum"=w1780) -> ()  [unwired: 2 in, 2 out]
            n824 = property on="中止编程模式 2" class="Bool (strict)"("DisabledEnum"=w1780) -> ()  [unwired: 2 in, 2 out]
          }
          frame False {
            w1807 = T3."Disabled and Grayed Out" ("禁用")
            w1815 = FALSE ("CAN状态")
            n825 = call "CAN_Init.vi"("设备类型"=w1822, "设备索引"=w1821, "波特率"=w1820, "CAN路数"=w1819, "操作类型"=enum16{"初始化CAN", "关闭CAN"}."关闭CAN", "滤波方式"=w1817, "IP"=w1814, "port"=w1812, "工作方式"=w1816, "PC端-协议类型"=w1813) -> ()  [unwired: 8 in, 2 out]
            n826 = local write "CAN状态"(w1815) -> ()
            n827 = local write "连接状态"(w1815) -> ()
            n828 = property on="手动进入编程模式" class="Bool (strict)"("DisabledEnum"=w1807) -> ()  [unwired: 2 in, 2 out]
            n829 = property on="中止编程模式" class="Bool (strict)"("DisabledEnum"=w1807) -> ()  [unwired: 2 in, 2 out]
            n830 = Concatenate Strings("" ("字符串"), "关闭CAN成功..." ("字符串"), "\n") -> (w1811:string)
            n831 = local write "Info："(w1811) -> ()
          }
        }
      }
      event "Info：": Shortcut Menu Selection (User) {
        n832 = event-data() -> ("ItemPath"=w1823:string)  [unwired: 1 in, 7 out]
        n833 = case shown="\"清空\"" w1823 {
          frame "假", Default {
          }
          frame "清空" {
            n834 = local write "Info："("" ("Info：")) -> ()
          }
        }
      }
      event Menu Selection (User) {
        n835 = event-data() -> ("ItemTag"=w1826:string)  [unwired: 1 in, 6 out]
        n836 = case shown="\"烧录多块\"" w1826 {
          tunnel: [FALSE ("Mode") TRUE ("Mode")] -> w1825
          frame "烧录多块" {
          }
          frame "烧录一块", Default {
          }
        }
        n837 = local write "Mode"(w1825) -> ()
      }
      event "类型": Value Change {
        n838 = event-data() -> ("NewVal"=w1830:u32)  [unwired: 1 in, 5 out]
        n839 = case shown="17" w1830 {
          tunnel: w1829 -> [_ w1834]
          frame 0, Default {
          }
          frame 17 {
            n840 = call "PortSet.vi"("error in (no error)"=w1834) -> ("PC端-协议类型 2"=→"PC端-协议类型 2":enum16{"TCP服务器Server", "TCP客户端Client"}, "通信端口:"=→"通信端口:":dbl, "CANET地址格式如：192.168.0.178"=→"CANET地址格式如：192.168.0.178":string)  [unwired: 7 in, 1 out]
          }
        }
      }
      event "类型": Mouse Down {
        w1835 = u16 4 items=["PCI5121"=1, "PCI9810"=2, "USBCAN1"=3, "USBCAN2"=4, "PCI9820"=5, "CAN232"=6, "PCI5110"=7, "CANLite(mini)"=8, "ISA9620"=9, "ISA5420"=10, "PC104CAN"=11, "CANET"=17, "DNP9810"=13] ("设备类型")
        n841 = event-data() -> ()  [unwired: 1 in, 8 out]
        n842 = local write "类型"(w1835) -> ()
      }
      event "Monitor": Value Change {
        n843 = event-data() -> ("NewVal"=w1839:bool)  [unwired: 1 in, 5 out]
        n844 = local read "板类型"() -> (w1838:enum16{"请选择板类型", "主板", "从板", "高压板"})
        n845 = Equal?(x=w1838, y=enum16{"请选择板类型", "主板", "从板", "高压板"}."请选择板类型") -> (x = y?=w1836:bool)
        n846 = case shown="True" w1836 {
          tunnel: w1839 -> [w1842 _]
          frame False {
            n847 = Select(t=0.0, s=w1842, f=2.0) -> (s? t:f=w1843:dbl)
            n848 = property on="手动进入编程模式" class="Bool (strict)"("Disabled"=w1843) -> ()  [unwired: 2 in, 2 out]
            "Monitor_flag" <- w1842
          }
          frame True {
            n849 = invoke on="Monitor" class="Bool" method="Reinit To Default"() -> ()  [unwired: 3 in, 3 out]
            n850 = One Button Dialog(message=" 请选择板的类型！！" ("消息")) -> ()  [unwired: 1 in, 1 out]
          }
        }
      }
      event "应用程序路径": Value Change {
        n851 = event-data() -> ("NewVal"=w1846:path)  [unwired: 1 in, 5 out]
        n852 = Not A Number/Path/Refnum?(number/path/refnum=w1846) -> (NaN/Path/Refnum?=w1849:bool)
        n853 = Strip Path(path=w1846) -> (name=w1845:string)  [unwired: 1 out]
        n854 = String Subset(string=w1845, offset (0)=6 ("偏移量(0)"), length (rest)=2 ("长度（剩余）")) -> (substring=w1850:string)
        n855 = case shown="\"SS\"" w1850 {
          tunnel: [TRUE ("y") FALSE ("y") FALSE ("y")] -> w1847
          frame "假", Default {
            n856 = local read "Info："() -> (w1854:string)
            n857 = Concatenate Strings(w1854, "无法识别板类型！\n" ("字符串")) -> (w1856:string)
            n858 = local write "Info："(w1856) -> ()
          }
          frame "MS" {
            n859 = local read "Info："() -> (w1858:string)
            n860 = local write "目标板类型"(enum16{"BCU/主板", "BMU/从板"}."BCU/主板" ("类型")) -> ()
            n861 = property on="请选择板号" class="Ring (strict)"("Visible"=FALSE ("可见")) -> ()  [unwired: 2 in, 2 out]
            n862 = Concatenate Strings(w1858, "通过文件识别为主板！\n" ("字符串")) -> (w1859:string)
            n863 = local write "Info："(w1859) -> ()
          }
          frame "SS" {
            n864 = local read "Info："() -> (w1864:string)
            n865 = local write "目标板类型"(enum16{"BCU/主板", "BMU/从板"}."BMU/从板" ("类型")) -> ()
            n866 = property on="请选择板号" class="Ring (strict)"("Visible"=TRUE ("可见")) -> ()  [unwired: 2 in, 2 out]
            n867 = Concatenate Strings(w1864, "通过文件识别为从板！\n" ("字符串")) -> (w1865:string)
            n868 = local write "Info："(w1865) -> ()
          }
        }
        n869 = Or(x=w1849, y=w1847) -> (x .or. y?=w1848:bool)
        n870 = case shown="False" w1848 {
          tunnel: w1846 -> [w1904 _]
          frame False {
            n871 = Path To String(path=w1904) -> (string=w1878:string)
            n872 = local read "Info："() -> (w1874:string)
            n873 = String Subset(string=w1878, offset (0)=6 ("偏移量(0)"), length (rest)=2 ("长度（剩余）")) -> (substring=w1875:string)
            n874 = call-poly <vilib>:"Read From Spreadsheet File.vi"("file path (dialog if empty)"=w1904) -> ("all rows"=w1906:string[][])  [unwired: 6 in, 4 out]
            n875 = call <vilib>:"Space Constant.vi"() -> ("String"=w1902:string)
            n876 = Search and Replace String(replace all?=TRUE ("替换全部？(F)"), input string=w1878, search string=w1902, replace string="" ("替换字符串(\"\")")) -> (result string=w1889:string)  [unwired: 4 in, 3 out]
            n877 = case shown="\"真\"" w1875 {
              frame "假", Default {
              }
              frame "真" {
              }
            }
            n878 = Concatenate Strings(w1874, "文件加载成功！\n" ("字符串")) -> (w1872:string)
            n879 = Index Array(array=w1906, index (col)=0 ("禁用的索引 (列)")) -> (element=w1893:string[])  [unwired: 1 in]
            n880 = Search/Split String(string=w1889, search string/char (-)="(MD5=" ("搜索字符串/字符(-)")) -> (match + rest of string=w1886:string, offset of match=w1896:i32)  [unwired: 1 in, 1 out]
            n881 = local write "Info："(w1872) -> ()
            n882 = Delete From Array(array=w1893, length=1 ("长度"), index=0 ("索引")) -> (array with subset deleted=w1885:string[])  [unwired: 1 out]
            n883 = call <vilib>:"MD5Checksum File.vi"("Path"=w1904) -> ("MD5 message-digest"=w1869:string)  [unwired: 9 in, 1 out]
            n884 = Array Size(array=w1885) -> (size(s)=w1883:i32)
            n885 = Decrement(x=w1883) -> (x-1=w1882:i32)
            n886 = Delete From Array(array=w1885, length=1 ("长度"), index=w1882) -> (array with subset deleted=w1880:string[])  [unwired: 1 out]
            n887 = Array Size(array=w1880) -> (size(s)=→"总行数":i32)
            n888 = local write "校验码实际值"(w1869) -> ()
            n889 = Add(x=w1896, y=5) -> (x+y=w1897:i32)
            n890 = Search/Split String(string=w1889, search string/char (-)=")" ("搜索字符串/字符(-)")) -> ()  [unwired: 1 in, 3 out]
            n891 = String Subset(string=w1886, offset (0)=45 ("偏移量(0)"), length (rest)=8 ("长度（剩余）")) -> ()  [unwired: 1 out]
            n892 = String Subset(string=w1889, offset (0)=w1897, length (rest)=32 ("长度（剩余）")) -> (substring=w1887:string)
            n893 = Equal?(x=w1887, y=w1869) -> (x = y?=w1894:bool)
            n894 = case shown="True" w1894 {
              frame False {
                n895 = Build Array(cluster{u32, u32} {16711680, 0}) -> (w1936:cluster{u32, u32}[])
                n896 = property on="MD5校验" class="Bool (strict)"("Colors [4]"=w1936, "BoolText.Text"="失败" ("布尔文本.文本")) -> ()  [unwired: 2 in, 2 out]
              }
              frame True {
                n897 = Build Array(cluster{u32, u32} {6618880, 0}) -> (w1939:cluster{u32, u32}[])
                n898 = property on="MD5校验" class="Bool (strict)"("Colors [4]"=w1939, "BoolText.Text"="成功" ("布尔文本.文本")) -> ()  [unwired: 2 in, 2 out]
              }
            }
            n899 = local write "校验码期望值"(w1887) -> ()
            n900 = for {
              tunnel: w1880 -> [w1917] mode=indexing
              shift-right: [w1915] -> w1870
              shift-left: u16 0 ("偏移量(0)") -> [w1916]
              tunnel: [w1909] -> w1871 mode=indexing
              n901 = String Subset(string=w1917, offset (0)=1 ("偏移量(0)"), length (rest)=1 ("长度（子字符串长度）")) -> (substring=w1920:string)
              n902 = case shown="\"1\", Default" w1920 {
                tunnel: ["01" ("子字符串(\"\")") "02" ("子字符串(\"\")")] -> w1921
                frame "1", Default {
                }
                frame "2" {
                }
              }
              n903 = String Subset(string=w1917, offset (0)=2 ("偏移量(0)")) -> (substring=w1923:string)  [unwired: 1 in]
              n904 = Concatenate Strings("FFFFFFFFFFFF" ("子字符串(\"\")"), w1921, w1923) -> (w1909:string)
              n905 = String Subset(string=w1909, offset (0)=12 ("偏移量(0)")) -> (substring=w1907:string)  [unwired: 1 in]
              n906 = String Length(string=w1907) -> (length=w1914:i32)
              n907 = Divide(x=w1914, y=2) -> (x/y=w1912:dbl)
              n908 = for {
                N: w1912 -> [_]
                tunnel: w1907 -> [w1932]
                shift-right: [w1927] -> w1910
                shift-left: u16 0 ("偏移量(0)") -> [w1925]
                i -> [w1931]
                w1929 = 2 ("x")
                n909 = Multiply(x=w1929, y=w1931) -> (x*y=w1930:i32)
                n910 = String Subset(string=w1932, offset (0)=w1930, length (rest)=w1929) -> (substring=w1928:string)
                n911 = call "ASCII_To_Hex.vi"("ASCII String"=w1928) -> ("hex1"=w1926:u8)  [unwired: 6 in, 4 out]
                n912 = Add(x=w1925, y=w1926) -> (x+y=w1927:u16)
              }
              n913 = Add(x=w1916, y=w1910) -> (x+y=w1915:u16)
            }
            n914 = local write "CRC16"(w1870) -> ()
            n915 = local write "子数组"(w1871) -> ()
          }
          frame True {
          }
        }
      }
      event "手动进入编程模式": Value Change {
        n916 = event-data() -> ("NewVal"=w1941:bool)  [unwired: 1 in, 5 out]
        n917 = case shown="True" w1941 {
          tunnel: w1942 -> [_ w1945]
          frame False {
          }
          frame True {
            n918 = Empty String/Path?(string/path="应用程序路径") -> (empty?=w1943:bool)
            n919 = case shown="False" w1943 {
              tunnel: w1945 -> [w1949 _]
              frame False {
                n920 = local write "update flag"(TRUE ("update flag")) -> ()
                n921 = Two Button Dialog(message="请确认需要下载的BMU编号正确！\nBMU正常上电！\n应用程序文件选择正确 !" ("消息")) -> (T button?=w1948:bool)  [unwired: 2 in]
                n922 = case shown="True" w1948 {
                  tunnel: w1949 -> [_ w1950]
                  frame False {
                  }
                  frame True {
                    n923 = stacked-sequence {
                      tunnel: w1950 -> [_ _ _]
                      frame #0 {
                        n924 = disable-structure shown="启用" {
                          frame Enabled {
                            n925 = local read "CAN路数"() -> (w1956:u32)
                            n926 = local read "设备索引"() -> (w1957:u32)
                            n927 = local read "类型"() -> (w1958:u32)
                            n928 = dll-call lib="PTH2{abs DPCTools2.sourceSNV-AutoTestV1.0.0ASettingsSEQEditDriver平台BCUAutoBurnSettingsControlCAN.dll" fn="VCI_ClearBuffer" label="VCI_Clearbuffer"(error in=errorcluster {"status"=FALSE, "code"=0, "source"=""} ("错误输入（无错误）"), "DeviceType"=w1958, "DeviceInd"=w1957, "CANInd"=w1956) -> (error out=→"错误输出 3":errorcluster)  [unwired: 3 in, 4 out]
                          }
                          frame Disabled {
                          }
                        }
                        n929 = local write "boot模式应答...成功"(FALSE) -> ()
                        "boot模式应答计数" <- 0
                        "进入烧录" <- TRUE ("布尔")
                      }
                      frame #1 {
                        w1964 = TRUE ("T1")
                        w1963 = TRUE ("T1")
                        n930 = Concatenate Strings("" ("字符串"), "boot模式请求..." ("字符串"), "\n") -> (w1962:string)
                        n931 = local write "Info："(w1962) -> ()
                        n932 = local write "T2"(w1963) -> ()
                        n933 = local write "T3"(w1964) -> ()
                        n934 = local write "T1"(w1963) -> ()
                        n935 = local write "T4"(w1964) -> ()
                        n936 = local write "T5"(w1964) -> ()
                        n937 = local write "T6"(w1964) -> ()
                        n938 = local write "T7"(w1964) -> ()
                        n939 = local write "T8"(u8 0 ("T8")) -> ()
                        n940 = local write "T9"(w1964) -> ()
                      }
                      frame #2 {
                        n941 = local read "目标板类型"() -> (w1967:enum16{"BCU/主板", "BMU/从板"})
                        n942 = case shown="\"BMU/从板\"" w1967 {
                          tunnel: [u16 0 ("请选择板号") w1980] -> w1968
                          frame "BCU/主板", Default {
                          }
                          frame "BMU/从板" {
                            n943 = local read "请选择板号"() -> (w1980:u16)
                          }
                        }
                        n944 = Tick Count (ms)() -> (millisecond timer value=→"start":u32)
                        n945 = Multiply(x=w1968, y=u16 256) -> (x*y=w1971:u16)
                        n946 = Add(x=u32 65681 ("ID"), y=w1971) -> (x+y=w1969:u32)
                        n947 = local read "VCI_CAN_OBJ_T"() -> (w1973:T2)
                        n948 = case shown="1, Default" w1968 {
                          tunnel: [w1985 w1997] -> w1977
                          tunnel: w1973 -> [w1984 w1996]
                          tunnel: w1969 -> [w1982 w1994]
                          frame 0 {
                            w1981 = u8 170
                            w1988 = u8 0 ("元素")
                            n949 = Bundle(cluster=w1984, "ID"=w1982, "TimeStamp"=u8 0 ("RemoteFlag"), "TimeFlag"=u8 1, "SendType"=u8 0 ("DataLen"), "RemoteFlag"=u8 0, "ExternFlag"=u8 1, "DataLen"=u8 8, u8 1 ("元素"), w1981, w1981, w1981, w1981, w1988, w1988, w1988) -> (w1985:T2)  [unwired: 3 in]
                          }
                          frame 1, Default {
                            w1993 = u8 187
                            w2000 = u8 0 ("元素")
                            n950 = Bundle(cluster=w1996, "ID"=w1994, "TimeStamp"=u8 0 ("RemoteFlag"), "TimeFlag"=u8 1, "SendType"=u8 0 ("DataLen"), "RemoteFlag"=u8 0, "ExternFlag"=u8 1, "DataLen"=u8 8, u8 1 ("元素"), w1993, w1993, w1993, w1993, w2000, w2000, w2000) -> (w1997:T2)  [unwired: 3 in]
                          }
                        }
                        n951 = local read "设备索引"() -> (w1975:u32)
                        n952 = local read "CAN路数"() -> (w1974:u32)
                        n953 = local read "类型"() -> (w1976:u32)
                        n954 = dll-call lib="PTH2{abs DPCTools2.sourceSNV-AutoTestV1.0.0ASettingsSEQEditDriver平台BCUAutoBurnSettingsControlCAN.dll" fn="VCI_Transmit"("DeviceType"=w1976, "DeviceInd"=w1975, "CANInd"=w1974, "pSend"=w1977, "Len"=u32 1) -> ()  [unwired: 5 in, 6 out]
                      }
                    }
                  }
                }
              }
              frame True {
                n955 = One Button Dialog(message="请先选择应用程序路径" ("消息")) -> ()  [unwired: 1 in, 1 out]
              }
            }
          }
        }
      }
      event "开始监控 2": Value Change {
        n956 = event-data() -> ("NewVal"=w2006:bool)  [unwired: 1 in, 5 out]
        n957 = local write "TEMP"(w2006) -> ()
      }
      event Panel Close? {
        n958 = event-data() -> ()  [unwired: 1 in, 4 out]
        n959 = local read "设备索引"() -> (w2009:u32)
        n960 = local read "CAN路数"() -> (w2011:u32)
        n961 = local read "波特率"() -> (w2010:T1)
        n962 = local read "滤波方式"() -> (w2012:u8)
        n963 = local read "工作方式"() -> (w2013:u8)
        n964 = local read "类型"() -> (w2008:u32)
        n965 = call "CAN_Init.vi"("设备类型"=w2008, "设备索引"=w2009, "波特率"=w2010, "CAN路数"=w2011, "操作类型"=enum16{"初始化CAN", "关闭CAN"}."关闭CAN", "滤波方式"=w2012, "工作方式"=w2013) -> ("error out"=w2007:errorcluster)  [unwired: 11 in, 1 out]
        n966 = flat-sequence {
          tunnel: w2007 -> [_]
          frame #0 {
            n967 = Quit LabVIEW(quit? (T)=TRUE ("退出？(T)")) -> ()
          }
        }
        n968 = event-data("Discard?"=TRUE ("放弃？")) -> ()  [unwired: 1 in, 1 out]
      }
    }
  }
  n969 = property on="手动进入编程模式" class="Bool (strict)"("DisabledEnum"=T3."Disabled and Grayed Out" ("禁用")) -> ()  [unwired: 2 in, 2 out]
  n970 = local write "开始下载数据"(FALSE ("开始下载数据")) -> ()
  n971 = Release Queue(queue=w3, error in (no error)=w2) -> ()  [unwired: 1 in, 3 out]
  n972 = local write "start"(u32 0 ("start")) -> ()
  n973 = Build Array(cluster{u32, u32} {0, 0}) -> (w27:cluster{u32, u32}[])
  n974 = local write "Info："("" ("字符串")) -> ()
  n975 = local write "进入烧录"(FALSE ("进入烧录")) -> ()
  n976 = property on="MD5校验" class="Bool (strict)"("Colors [4]"=w27, "BoolText.Text"="失败" ("布尔文本.文本")) -> ()  [unwired: 2 in, 2 out]
  n977 = local write "子数组"(string[] ["  "] ("子数组")) -> ()
  n978 = local write "发送数据长度"(0.0 ("发送数据长度")) -> ()
  n979 = local write "擦除完成"(w37) -> ()
  n980 = local write "进入烧录模式"(w37) -> ()
  "连接状态" <- FALSE ("CAN连接状态")
  "CAN数据" <- FALSE ("烧录中")
  "进度" <- u8 0 ("进度")
  "烧录结果" <- FALSE ("烧录完成")
  "Mode" <- TRUE ("Mode")
  "update flag" <- FALSE
